vi "Periodic Tasks.vi"(8 "error in":errorcluster) -> ()   [LabVIEW 2015]
doc: "This VI runs in parallel to other tasks. It can contain as many user-defined periodic loops as you need. These can carry out PID or other sorts of timed response."
uses:
  <vilib>/Rock Robotics/WPI/PWM/Servo/WPI_ServoDeviceRef.ctl
  <vilib>/Rock Robotics/SystemInterfaces/DIO/FPGA_DIOPWMChannel.ctl
  <vilib>/Rock Robotics/WPI/PWM/WPI_PWMDeadband.ctl
  Team Code/IMU/LSM9DS1DevRef.ctl
  <vilib>/Rock Robotics/SystemInterfaces/i2clib/i2c_bus.ctl
  Team Code/IMU/Gyro_TypeDef.ctl
  Team Code/IMU/Accel_TypeDef.ctl
  Team Code/IMU/Mag_TypeDef.ctl
  Team Code/Periodic Task/Intake Enum..ctl
  Team Code/Periodic Task/Arm_defense_Type_Def.ctl
  Team Code/Periodic Task/Motor_Dir_Type_Def.ctl
  <vilib>/Rock Robotics/WPI/Solenoid/WPI_SolenoidValue.ctl
  <vilib>/Rock Robotics/WPI/MotorControl/WPI_MotorControlDeviceRef.ctl
  <vilib>/Rock Robotics/WPI/MotorControl/WPI_MotorControlType.ctl
  <vilib>/Rock Robotics/WPI/CAN/Jaguar/SubVIs/WPI_CANJaguar_ControlMode.ctl
  <vilib>/Rock Robotics/WPI/CAN/TalonSRX/WPI_CANTalonSRX_APIControlMode.ctl
  <vilib>/Rock Robotics/WPI/Solenoid/WPI_SolenoidDevRef.ctl
  <vilib>/Rock Robotics/WPI/Solenoid/WPI_SolenoidChannel.ctl
  Team Code/IMU/IMU_Global.vi
  Team Code/Global_Var/Drive_Global.vi
panel:
  out "Pitch":cluster{dbl, "Out":dbl, "Out":dbl}(graph)
  in  "Pitch_FIlt":dbl=0.1
  out "Waveform Chart":cluster{"Yaw":dbl, "Angle":dbl}(graph)
  in  "Quick_Turn":bool=TRUE
  in  "Reset":bool
  in  "PID Gains":T1
  in  "Drive_En_Reset":bool
  in  "auto_ds_en":bool
  in  "auto_us_en":bool
  in  "auto_us_spd":dbl=60000.0
  in  "auto_ds_spd_hiload":dbl
  in  "low_throt_thresh":dbl=20.0 format="%#_13g"
  in  "high_throt_thresh":dbl=75.0 format="%#_13g"
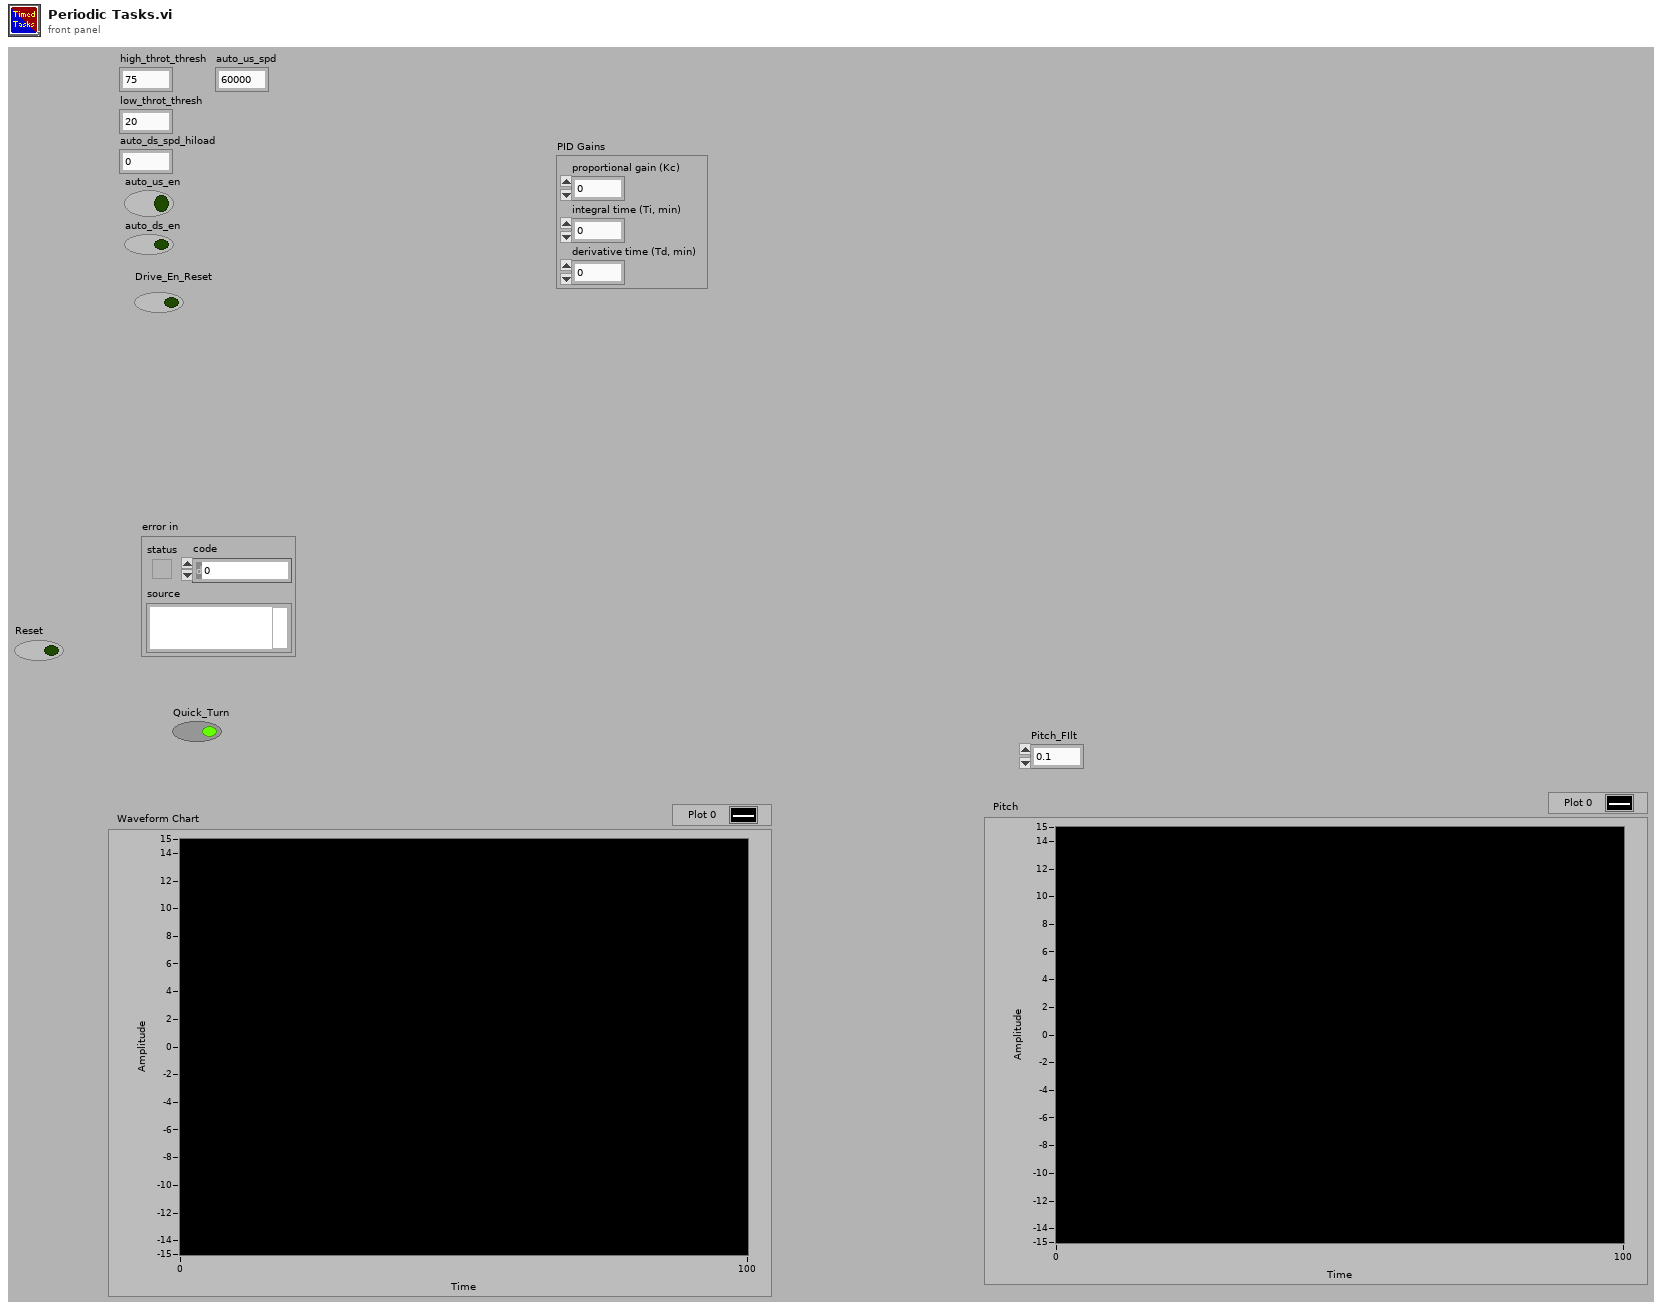
[diagram p1: front panel]
types:
  T1 = cluster{"proportional gain (Kc)":dbl, "integral time (Ti, min)":dbl, "derivative time (Td, min)":dbl}
  T2 = typedef "WPI_ServoDeviceRef.ctl" = cluster{"DeviceStatus":errorcluster, "PWM Channel":T3, "DeadBand":T4}
  T3 = typedef "FPGA_DIOPWMChannel.ctl" = enum8{"PWM 0", "PWM 1", "PWM 2", "PWM 3", "PWM 4", "PWM 5", "PWM 6", "PWM 7", "PWM 8", "PWM 9", "PWM MXP 0", "PWM MXP 1", "PWM MXP 2", "PWM MXP 3", "PWM MXP 4", "PWM MXP 5", "PWM MXP 6", "PWM MXP 7", "PWM MXP 8", "PWM MXP 9", "Invalid"}
  T4 = typedef "WPI_PWMDeadband.ctl" = cluster{"Name":string, "maxPositivePwm":i32, "minPositivePwm":i32, "centerPwm":i32, "maxNegativePwm":i32, "minNegativePwm":i32, "angularRange":u16}
  T5 = cluster{"ServoDeviceRef":T2, "error out":errorcluster}
  T6 = typedef "Motor_Type_Def.ctl" = cluster{"Drive_Motor":cluster{"RobotDriveDevRef":T7, "error out":errorcluster}, "Intake_1":cluster{"MotorControlDevRef":T8, "error out":errorcluster}, "Intake_Stage":cluster{"MotorControlDevRef":T8, "error out":errorcluster}, "Shooter_Motor_1":cluster{"MotorControlDevRef":T8, "error out":errorcluster}}
  T7 = typedef "WPI_RobotDriveDevRef.ctl" = cluster{"DevStatus":errorcluster, "Motors[]":T8[], "Square Inputs":bool, "Max Output":dbl}
  T8 = typedef "WPI_MotorControlDeviceRef.ctl" = cluster{"DeviceStatus":errorcluster, "Type":T9, "PWM":cluster{"PWM Channel":T3, "DeadBand":T4}, "CAN":cluster{"Device Number":u8, "Control Mode":T10, "Semaphore":T11, "Max Vout":dbl, "TalonSRX Control Mode":T12}, "Invert":bool}
  T9 = typedef "WPI_MotorControlType.ctl" = enum16{"PWM", "CAN", "CANTalonSRX"}
  T10 = typedef "WPI_CANJaguar_ControlMode.ctl" = enum8{"Percent VBus", "Current", "Speed", "Position", "Voltage"}
  T11 = typedef "Semaphore RefNum" = refnum<k1>
  T12 = typedef "WPI_CANTalonSRX_APIControlMode.ctl" = enum8{"Percent VBus", "Speed", "Position", "Slave", "Unchanged / Invalid", "Voltage Compensation", "Current", "Motion Profile"}
  T13 = typedef "Pneu_Type_Def.ctl" = cluster{"Intake_Arm":cluster{"SolenoidDevRef":T14, "error out":errorcluster}, "Gear":cluster{"SolenoidDevRef":T14, "error out":errorcluster}, "Flipper":cluster{"SolenoidDevRef":T14, "error out":errorcluster}, "Arm_defense":cluster{"SolenoidDevRef":T14, "error out":errorcluster}, "Compressor":cluster{"CompressorDevRef":T16, "error out":errorcluster}}
  T14 = typedef "WPI_SolenoidDevRef.ctl" = cluster{"DevStatus":errorcluster, "Pneumatics Control Module":u8, "Forward Solenoid Channel":T15, "Reverse Solenoid Channel":T15}
  T15 = typedef "WPI_SolenoidChannel.ctl" = enum8{"Solenoid 0", "Solenoid 1", "Solenoid 2", "Solenoid 3", "Solenoid 4", "Solenoid 5", "Solenoid 6", "Solenoid 7", "Invalid"}
  T16 = typedef "WPI_CompressorDevRef.ctl" = cluster{"DevStatus":errorcluster, "Pneumatics Control Module":u8}
  T17 = typedef "DIO_Type_Def.ctl" = cluster{"Left_Back":cluster{"SonarMB1010DigitalDevRef":T18, "error out":errorcluster}, "Left_Front":cluster{"SonarMB1010DigitalDevRef":T18, "error out":errorcluster}, "Right_Back":cluster{"SonarMB1010DigitalDevRef":T18, "error out":errorcluster}, "Right_Front":cluster{"SonarMB1010DigitalDevRef":T18, "error out":errorcluster}, "Front":cluster{"SonarMB1010DigitalDevRef":T18, "error out":errorcluster}, "Left Encoder":cluster{"EncoderDevRef":T21, "error out":errorcluster}, "Right Encoder":cluster{"EncoderDevRef":T21, "error out":errorcluster}, "Shooter Encoder":cluster{"CounterDevRef":T19, "error out":errorcluster}, "Intake_Storing":cluster{"DigitalInputDevRef":T24, "error out":errorcluster}, "Intake_Staged":cluster{"DigitalInputDevRef":T24, "error out":errorcluster}}
  T18 = typedef "WPI_SonarMB1010DigitalDeviceRef.ctl" = cluster{"CounterDevRef":T19, "Scaling factor (s/in)":dbl}
  T19 = typedef "WPI_CounterDevRef.ctl" = cluster{"DevStatus":errorcluster, "CntIndex":T20}
  T20 = typedef "FPGA_CounterCtrSystemIndex.ctl" = enum8{"Ctr 0", "Ctr 1", "Ctr 2", "Ctr 3", "Ctr 4", "Ctr 5", "Ctr 6", "Ctr 7", "Invalid"}
  T21 = typedef "WPI_EncoderDevRef.ctl" = cluster{"DevStatus":errorcluster, "EncoderIndex":T22, "CounterIndex":T20, "DistancePerCount":dbl, "Decoding Type":T23}
  T22 = typedef "FPGA_EncoderIdx.ctl" = enum8{"Enc 0", "Enc 1", "Enc 2", "Enc 3", "Enc 4", "Enc 5", "Enc 6", "Enc 7", "Invalid"}
  T23 = typedef "WPI_EncoderType.ctl" = enum16{"1x", "2x", "4x"}
  T24 = typedef "WPI_DigitalInputDevRef.ctl" = cluster{"DevStatus":errorcluster, "DIO Channel":T25}
  T25 = typedef "FPGA_DIOChannel.ctl" = enum8{"DIO 0", "DIO 1", "DIO 2", "DIO 3", "DIO 4", "DIO 5", "DIO 6", "DIO 7", "DIO 8", "DIO 9", "DIO MXP 0", "DIO MXP 1", "DIO MXP 2", "DIO MXP 3", "DIO MXP 4", "DIO MXP 5", "DIO MXP 6", "DIO MXP 7", "DIO MXP 8", "DIO MXP 9", "DIO MXP 10", "DIO MXP 11", "DIO MXP 12", "DIO MXP 13", "DIO MXP 14", "DIO MXP 15", "Invalid"}
  T26 = typedef "LSM9DS1DevRef.ctl" = cluster{"DevStatus":errorcluster, "Gyro Offset":cluster{"Xzero":dbl, "Yzero":dbl, "Zzero":dbl}, "StdDev Rates":cluster{"Xsdo":dbl, "Ysdo":dbl, "Zsdo":dbl}, "Reset":bool, "Accel Offset":cluster{"Xzero":dbl, "Yzero":dbl, "Zzero":dbl}, "Motion Thresh":dbl, "Mag Offset":cluster{"Xzero":dbl, "Yzero":dbl, "Zzero":dbl}, "I2C Bus":T27, "Handle":i32, "Anomaly Thresh":dbl, "Local Mag":dbl, "Accel/Gyro_Address":enum8{"0x6A", "0x6B"}, "Accel_Range":enum16{"±2g", "±16g", "±4g", "±8g", "disabled"}, "Gyro_Range":enum16{"±245dps", "±500dps", "disabled", "±2000dps"}, "Mag_Range":enum16{"±2 gauss", "±4 gauss", "±8 gauss", "±16 gauss", "disabled"}, "Mag_Address":enum8{"0x1C", "0x1E"}, "accel_active":bool, "gyro_active":bool, "mag_active":bool}
  T27 = typedef "i2c_bus.ctl" = enum16{"I2C On-Board", "I2C MXP", "Invalid"}
  T28 = typedef "WPI_GyroDevRef.ctl" = cluster{"DevStatus":errorcluster, "Analog Channel":T29, "Offset":dbl, "Gain (VoltsPerDegree/Second)":dbl, "Gyro Type":enum16{"Analog", "XRS450"}, "Handle":i32, "SPI Bus":T30, "Device Found":bool, "Sample Rate":dbl, "Calibrate On Open":bool}
  T29 = typedef "FPGA_AIChannel.ctl" = enum8{"AI 0", "AI 1", "AI 2", "AI 3", "AI MXP 0", "AI MXP 1", "AI MXP 2", "AI MXP 3", "Invalid"}
  T30 = typedef "spi_bus.ctl" = enum16{"SPI On-Board, CS0", "SPI On-Board, CS1", "SPI On-Board, CS2", "SPI On-Board, CS3", "SPI MXP", "Invalid"}
  T31 = typedef "WPI_AccelerometerDevRef.ctl" = cluster{"DevStatus":errorcluster, "Scaling":T32, "Analog Channels":T33, "I2C Bus":T27, "SPI Bus":T30, "Accel Range":T34, "ADXL Axes":T35, "Handle":i32, "Device Address":u8, "Accel Type":enum16{"Analog", "ADXL345 I2C", "ADXL345 SPI", "Internal", "ADXL362 SPI"}}
  T32 = typedef "WPI_AccelerometerScaling.ctl" = cluster{"Gain (VoltsPerG)":dbl, "Center Voltage":dbl}
  T33 = typedef "WPI_AccelerometerAnalogChannels.ctl" = cluster{"X-Axis":T29, "Y-Axis":T29, "Z-Axis":T29}
  T34 = typedef "ADXL345 Range.ctl" = u8
  T35 = typedef "WPI_AccelerometerADXL345 Axes.ctl" = cluster{"X-Axis":bool, "Y-Axis":bool, "Z-Axis":bool}
  T36 = cluster{"Auto_Aim":bool, "Auto_Aim_Enable":bool, "Shoot":bool, "Far_Shoot":bool}
  T37 = cluster{"Intake Arm Lowered":bool, "Motor Speed":dbl, "Rest_Encoder":bool, "Rest_Gyro":bool, "TeeterTotter Enable":bool, "Completed_Auto":bool}
  T38 = cluster{"Intake Arm Lowered":bool, "Motor Speed":dbl, "PortCullis_Enable":bool, "Rest_Encoder":bool, "Rest_Gyro":bool, "Completed_Auto":bool}
  T39 = cluster{"Motor Speed":dbl, "Rest_Encoder":bool, "Rest_Gyro":bool, "Rough Terrain On":bool, "Intake Arm Lowered":bool, "Completed_Auto":bool}
  T40 = cluster{"Drive_Enable":bool, "Auto_Aim":bool, "Intake Arm Lowered":bool, "Drive_FWD Speed":dbl, "One_Ball_Auto":bool, "Rest_Encoder":bool, "Rest_Gyro":bool, "Shoot":bool, "Stage":bool, "Angle_Setpoint":dbl}
  T41 = cluster{"Vision Distance":cluster{"1":dbl, "2":dbl, "3":dbl}, "Vision_angle":cluster{"1":dbl, "2":dbl, "3":dbl}, "Aimed?":bool}
  T42 = cluster{"Auto_Aim_Enable":bool, "CAM_Reset_IMU":bool, "Set_Point":dbl, "Aimed?":bool, "Enable_Cam":bool}
  T43 = typedef "Gyro_TypeDef.ctl" = cluster{"Pitch":dbl, "Yaw":dbl, "X Ang Rate":dbl, "Y Ang Rate":dbl, "Z Ang Rate":dbl, "Roll":dbl}
  T44 = typedef "Accel_TypeDef.ctl" = cluster{"X Accel":dbl, "Y Accel":dbl, "Z Accel":dbl, "Pitch":dbl, "Roll":dbl}
  T45 = typedef "Mag_TypeDef.ctl" = cluster{"X Mag":dbl, "Y Mag":dbl, "Z Mag":dbl}
  T46 = cluster{"LSM9DS1DevRef Out":T26, "Gyro":T43, "Accel":T44, "Mag":T45, "error out":errorcluster}
  T47 = cluster{"X-Axis":dbl, "Y-Axis":dbl, "Z-Axis":dbl}
  T48 = cluster{"Left_Back_Dist":dbl, "Left_Front_Dist":dbl, "Right_Back_Dist":dbl, "Right_Front_Dist":dbl, "Front_Dist":dbl, "Left_Dist":dbl, "Left_Angle":dbl, "Right_Dist":dbl, "Right_Angle":dbl}
  T49 = typedef "Auto_Selection.ctl" = enum16{"Low Bar", "Rough Terrain", "Rock Wall", "Ramparts", "Moat", "Cheval de Frise", "Portcullis", "None", "One  Ball", "Shoot"}
  T50 = cluster{"Auto_Selection":T49, "Auto_Enable":bool}
  T51 = cluster{"Right_En":cluster{"Distance":dbl, "Direction":bool, "Rate":dbl, "Stopped":bool}, "Left_En":cluster{"Distance":dbl, "Direction":bool, "Rate":dbl, "Stopped":bool}, "Shooter_En":cluster{"Distance":dbl, "Direction":bool, "Rate":dbl, "Stopped":bool}}
  T52 = typedef "WPI_DriverStationRobotMode2.ctl" = enum16{"Autonomous Disabled", "Autonomous Enabled", "Teleop Disabled", "Teleop Enabled", "Disconnected", "Finish", "Test Disabled", "Test Enabled", "Emergency Stopped"}
  T53 = typedef "WPI_CameraImageSize.ctl" = enum16{"640x480", "320x240", "160x120", "Custom"}
  T54 = cluster{"Climb":bool, "Close_Shot":bool, "Enable Vision":bool, "Far_Shot":bool, "Gear_Toggle":bool, "Intake":bool, "Left_Joystick_X":dbl, "Left_Joystick_Y":dbl, "Portcullis":bool, "Right_Joystick_X":dbl, "Right_Joystick_Y":dbl, "Robot Mode":T52, "image size":T53, "Speed Toggle":bool, "Intake Stage":bool, "Cheval":bool, "Intake_Motor_Man":dbl, "Stage_Motor_Man":dbl, "Lower_Intake_Arm":bool, "Lower_Intake_Def":bool, "Raise_Intake_Arm":bool, "Raise_Intake_Def":bool, "Flipper_Man":bool, "Auto_Aim":bool, "Low_Goal":bool}
  T55 = cluster{"Encoder_Var":cluster{"Right_En":cluster{"Distance":dbl, "Direction":bool, "Rate":dbl, "Stopped":bool}, "Left_En":cluster{"Distance":dbl, "Direction":bool, "Rate":dbl, "Stopped":bool}, "Shooter_En":cluster{"Distance":dbl, "Direction":bool, "Rate":dbl, "Stopped":bool}}, "JoyStick":cluster{"Climb":bool, "Close_Shot":bool, "Enable Vision":bool, "Far_Shot":bool, "Gear_Toggle":bool, "Intake":bool, "Left_Joystick_X":dbl, "Left_Joystick_Y":dbl, "Portcullis":bool, "Right_Joystick_X":dbl, "Right_Joystick_Y":dbl, "Robot Mode":T52, "image size":T53, "Speed Toggle":bool, "Intake Stage":bool, "Cheval":bool, "Intake_Motor_Man":dbl, "Stage_Motor_Man":dbl, "Lower_Intake_Arm":bool, "Lower_Intake_Def":bool, "Raise_Intake_Arm":bool, "Raise_Intake_Def":bool, "Flipper_Man":bool, "Auto_Aim":bool, "Low_Goal":bool}, "IMU":cluster{"LSM9DS1DevRef Out":T26, "Gyro":T43, "Accel":T44, "Mag":T45, "error out":errorcluster}, "Feedback":cluster{"Vision Distance":cluster{"1":dbl, "2":dbl, "3":dbl}, "Vision_angle":cluster{"1":dbl, "2":dbl, "3":dbl}, "Aimed?":bool}, "Ultar_Sonic":cluster{"Left_Back_Dist":dbl, "Left_Front_Dist":dbl, "Right_Back_Dist":dbl, "Right_Front_Dist":dbl, "Front_Dist":dbl, "Left_Dist":dbl, "Left_Angle":dbl, "Right_Dist":dbl, "Right_Angle":dbl}, "Auto_Contorl":cluster{"Auto_Selection":T49, "Auto_Enable":bool}}
  T56 = cluster{"Encoder_Var":cluster{"Right_En":cluster{"Distance":dbl, "Direction":bool, "Rate":dbl, "Stopped":bool}, "Left_En":cluster{"Distance":dbl, "Direction":bool, "Rate":dbl, "Stopped":bool}, "Shooter_En":cluster{"Distance":dbl, "Direction":bool, "Rate":dbl, "Stopped":bool}}, "JoyStick":cluster{"Climb":bool, "Close_Shot":bool, "Enable Vision":bool, "Far_Shot":bool, "Gear_Toggle":bool, "Intake":bool, "Left_Joystick_X":dbl, "Left_Joystick_Y":dbl, "Portcullis":bool, "Right_Joystick_X":dbl, "Right_Joystick_Y":dbl, "Robot Mode":T52, "image size":T53, "Speed Toggle":bool, "Intake Stage":bool, "Cheval":bool, "Intake_Motor_Man":dbl, "Stage_Motor_Man":dbl, "Lower_Intake_Arm":bool, "Lower_Intake_Def":bool, "Raise_Intake_Arm":bool, "Raise_Intake_Def":bool, "Flipper_Man":bool, "Auto_Aim":bool, "Low_Goal":bool}, "IMU":cluster{"LSM9DS1DevRef Out":T26, "Gyro":T43, "Accel":T44, "Mag":T45, "error out":errorcluster}, "Feedback":cluster{"Vision Distance":cluster{"1":dbl, "2":dbl, "3":dbl}, "Vision_angle":cluster{"1":dbl, "2":dbl, "3":dbl}, "Aimed?":bool}, "Ultar_Sonic":cluster{"Left_Back_Dist":dbl, "Left_Front_Dist":dbl, "Right_Back_Dist":dbl, "Right_Front_Dist":dbl, "Front_Dist":dbl, "Left_Dist":dbl, "Left_Angle":dbl, "Right_Dist":dbl, "Right_Angle":dbl}, "Rought_Ter":cluster{"Motor Speed":dbl, "Rest_Encoder":bool, "Rest_Gyro":bool, "Rough Terrain On":bool, "Intake Arm Lowered":bool, "Completed_Auto":bool}, "Portcullis":cluster{"Intake Arm Lowered":bool, "Motor Speed":dbl, "PortCullis_Enable":bool, "Rest_Encoder":bool, "Rest_Gyro":bool, "Completed_Auto":bool}, "One_Ball_Auto":cluster{"Drive_Enable":bool, "Auto_Aim":bool, "Intake Arm Lowered":bool, "Drive_FWD Speed":dbl, "One_Ball_Auto":bool, "Rest_Encoder":bool, "Rest_Gyro":bool, "Shoot":bool, "Stage":bool, "Angle_Setpoint":dbl}, "Teeter_Toter":cluster{"Intake Arm Lowered":bool, "Motor Speed":dbl, "Rest_Encoder":bool, "Rest_Gyro":bool, "TeeterTotter Enable":bool, "Completed_Auto":bool}, "Auto_Shoot":cluster{"Auto_Aim":bool, "Auto_Aim_Enable":bool, "Shoot":bool, "Far_Shoot":bool}}
  T57 = cluster{"Encoder_Var":cluster{"Right_En":cluster{"Distance":dbl, "Direction":bool, "Rate":dbl, "Stopped":bool}, "Left_En":cluster{"Distance":dbl, "Direction":bool, "Rate":dbl, "Stopped":bool}, "Shooter_En":cluster{"Distance":dbl, "Direction":bool, "Rate":dbl, "Stopped":bool}}, "JoyStick":cluster{"Climb":bool, "Close_Shot":bool, "Enable Vision":bool, "Far_Shot":bool, "Gear_Toggle":bool, "Intake":bool, "Left_Joystick_X":dbl, "Left_Joystick_Y":dbl, "Portcullis":bool, "Right_Joystick_X":dbl, "Right_Joystick_Y":dbl, "Robot Mode":T52, "image size":T53, "Speed Toggle":bool, "Intake Stage":bool, "Cheval":bool, "Intake_Motor_Man":dbl, "Stage_Motor_Man":dbl, "Lower_Intake_Arm":bool, "Lower_Intake_Def":bool, "Raise_Intake_Arm":bool, "Raise_Intake_Def":bool, "Flipper_Man":bool, "Auto_Aim":bool, "Low_Goal":bool}, "IMU":cluster{"LSM9DS1DevRef Out":T26, "Gyro":T43, "Accel":T44, "Mag":T45, "error out":errorcluster}, "Feedback":cluster{"Vision Distance":cluster{"1":dbl, "2":dbl, "3":dbl}, "Vision_angle":cluster{"1":dbl, "2":dbl, "3":dbl}, "Aimed?":bool}, "Ultar_Sonic":cluster{"Left_Back_Dist":dbl, "Left_Front_Dist":dbl, "Right_Back_Dist":dbl, "Right_Front_Dist":dbl, "Front_Dist":dbl, "Left_Dist":dbl, "Left_Angle":dbl, "Right_Dist":dbl, "Right_Angle":dbl}, "Rought_Ter":cluster{"Motor Speed":dbl, "Rest_Encoder":bool, "Rest_Gyro":bool, "Rough Terrain On":bool, "Intake Arm Lowered":bool, "Completed_Auto":bool}, "Portcullis":cluster{"Intake Arm Lowered":bool, "Motor Speed":dbl, "PortCullis_Enable":bool, "Rest_Encoder":bool, "Rest_Gyro":bool, "Completed_Auto":bool}, "One_Ball_Auto":cluster{"Drive_Enable":bool, "Auto_Aim":bool, "Intake Arm Lowered":bool, "Drive_FWD Speed":dbl, "One_Ball_Auto":bool, "Rest_Encoder":bool, "Rest_Gyro":bool, "Shoot":bool, "Stage":bool, "Angle_Setpoint":dbl}, "Teeter_Toter":cluster{"Intake Arm Lowered":bool, "Motor Speed":dbl, "Rest_Encoder":bool, "Rest_Gyro":bool, "TeeterTotter Enable":bool, "Completed_Auto":bool}, "AIM_Brain":cluster{"Auto_Aim_Enable":bool, "CAM_Reset_IMU":bool, "Set_Point":dbl, "Aimed?":bool, "Enable_Cam":bool}, "Auto_Shoot":cluster{"Auto_Aim":bool, "Auto_Aim_Enable":bool, "Shoot":bool, "Far_Shoot":bool}}
  T58 = cluster{"Encoder_Var":cluster{"Right_En":cluster{"Distance":dbl, "Direction":bool, "Rate":dbl, "Stopped":bool}, "Left_En":cluster{"Distance":dbl, "Direction":bool, "Rate":dbl, "Stopped":bool}, "Shooter_En":cluster{"Distance":dbl, "Direction":bool, "Rate":dbl, "Stopped":bool}}, "JoyStick":cluster{"Climb":bool, "Close_Shot":bool, "Enable Vision":bool, "Far_Shot":bool, "Gear_Toggle":bool, "Intake":bool, "Left_Joystick_X":dbl, "Left_Joystick_Y":dbl, "Portcullis":bool, "Right_Joystick_X":dbl, "Right_Joystick_Y":dbl, "Robot Mode":T52, "image size":T53, "Speed Toggle":bool, "Intake Stage":bool, "Cheval":bool, "Intake_Motor_Man":dbl, "Stage_Motor_Man":dbl, "Lower_Intake_Arm":bool, "Lower_Intake_Def":bool, "Raise_Intake_Arm":bool, "Raise_Intake_Def":bool, "Flipper_Man":bool, "Auto_Aim":bool, "Low_Goal":bool}, "IMU":cluster{"LSM9DS1DevRef Out":T26, "Gyro":T43, "Accel":T44, "Mag":T45, "error out":errorcluster}, "Feedback":cluster{"Vision Distance":cluster{"1":dbl, "2":dbl, "3":dbl}, "Vision_angle":cluster{"1":dbl, "2":dbl, "3":dbl}, "Aimed?":bool}, "Ultar_Sonic":cluster{"Left_Back_Dist":dbl, "Left_Front_Dist":dbl, "Right_Back_Dist":dbl, "Right_Front_Dist":dbl, "Front_Dist":dbl, "Left_Dist":dbl, "Left_Angle":dbl, "Right_Dist":dbl, "Right_Angle":dbl}, "Rought_Ter":cluster{"Motor Speed":dbl, "Rest_Encoder":bool, "Rest_Gyro":bool, "Rough Terrain On":bool, "Intake Arm Lowered":bool, "Completed_Auto":bool}, "Portcullis":cluster{"Intake Arm Lowered":bool, "Motor Speed":dbl, "PortCullis_Enable":bool, "Rest_Encoder":bool, "Rest_Gyro":bool, "Completed_Auto":bool}, "One_Ball_Auto":cluster{"Drive_Enable":bool, "Auto_Aim":bool, "Intake Arm Lowered":bool, "Drive_FWD Speed":dbl, "One_Ball_Auto":bool, "Rest_Encoder":bool, "Rest_Gyro":bool, "Shoot":bool, "Stage":bool, "Angle_Setpoint":dbl}, "Teeter_Toter":cluster{"Intake Arm Lowered":bool, "Motor Speed":dbl, "Rest_Encoder":bool, "Rest_Gyro":bool, "TeeterTotter Enable":bool, "Completed_Auto":bool}, "AIM_Brain":cluster{"Auto_Aim_Enable":bool, "CAM_Reset_IMU":bool, "Set_Point":dbl, "Aimed?":bool, "Enable_Cam":bool}, "Gear_Brain":cluster{"High_Gear_Cmd":bool}, "Setpoint_Arb":cluster{"Any True?":bool, "P Out":dbl}, "Drive":cluster{"Any True?":bool, "P Out":dbl}, "Auto_Shoot":cluster{"Auto_Aim":bool, "Auto_Aim_Enable":bool, "Shoot":bool, "Far_Shoot":bool}}
  T59 = cluster{"Climb_Motor_1":T8, "Climb_Motor_2":T8, "Climb_Pneu":T14}
  T60 = typedef "Arm_defense_Type_Def.ctl" = enum16{"Cheval de Frise", "Portcullis", "Out", "In", "Ball_Pickup"}
  T61 = typedef "WPI_SolenoidValue.ctl" = enum16{"Off", "On", "Forward", "Reverse"}
  T62 = cluster{"Gear Co mmand":T61, "Intake_Arm":T61, "Shooter_Arm":T61, "Flipper":T61}
  T63 = typedef "Motor_Dir_Type_Def.ctl" = enum16{"In", "Out", "Off"}
  T64 = cluster{"Shooter_Active":bool, "Stage_Motor":T63, "Shooter_Motor":dbl, "Shooter_Arm":T60}
  T65 = typedef "Intake Enum..ctl" = enum16{"Float", "Intake Portcullis", "Intake Ball Pickup", "Intake Cheval", " Intake Raised"}
  T66 = cluster{"Intake_Arm_Man_Act":bool, "Intake_Def_Man":T60, "Intake_Def_Man_Act":bool, "Intake_Motor_Man":T63, "Intake_Motor_Man_Act":bool, "Stage_Motor_Man":T63, "Stage_Motor_Man_Act":bool, "Flipper_Man":enum16{"Closed", "Open"}, "Flipper_Man_Act":bool, "Intake_Arm_Man":T65}
  T67 = cluster{"Intake_Motor_CMD":dbl, "Stage_Motor_CMD":dbl}
  T68 = cluster{"Intake Motor":T63, "Stage Motor":T63, "Flipper":enum16{"Closed", "Open"}, "Stage_Active":bool}
  T69 = cluster{"Intake_Motor":T63, "Intake_Position":T65, "Stage_Motor":T63, "Arm_Defense":T60, "Flipper":enum16{"Closed", "Open"}, "Intake_Active":bool}
  T70 = cluster{"Any True?":bool, "P_Out":enum16{"Closed", "Open"}}
  T71 = cluster{"Intake_Pos":T65, "Cheval_Active":bool, "Arm_Defense":T60}
  T72 = cluster{"Arm_Defense":T60, "Intake_Pos":T65, "Portcullis Active":bool}
  T73 = cluster{"Intake Storing":bool, "Intake_Stage":bool}
  T74 = cluster{"Ref_Num":cluster{"Motor":T6, "Pneu":T13, "DIO":T17}, "Ultar_Sonic":cluster{"Left_Back_Dist":dbl, "Left_Front_Dist":dbl, "Right_Back_Dist":dbl, "Right_Front_Dist":dbl, "Front_Dist":dbl, "Left_Dist":dbl, "Left_Angle":dbl, "Right_Dist":dbl, "Right_Angle":dbl}, "JoyStick":cluster{"Climb":bool, "Close_Shot":bool, "Enable Vision":bool, "Far_Shot":bool, "Gear_Toggle":bool, "Intake":bool, "Left_Joystick_X":dbl, "Left_Joystick_Y":dbl, "Portcullis":bool, "Right_Joystick_X":dbl, "Right_Joystick_Y":dbl, "Robot Mode":T52, "image size":T53, "Speed Toggle":bool, "Intake Stage":bool, "Cheval":bool, "Intake_Motor_Man":dbl, "Stage_Motor_Man":dbl, "Lower_Intake_Arm":bool, "Lower_Intake_Def":bool, "Raise_Intake_Arm":bool, "Raise_Intake_Def":bool, "Flipper_Man":bool, "Auto_Aim":bool, "Low_Goal":bool}, "Intake Var":cluster{"Intake Storing":bool, "Intake_Stage":bool}}
  T75 = cluster{"Ref_Num":cluster{"Motor":T6, "Pneu":T13, "DIO":T17}, "Ultar_Sonic":cluster{"Left_Back_Dist":dbl, "Left_Front_Dist":dbl, "Right_Back_Dist":dbl, "Right_Front_Dist":dbl, "Front_Dist":dbl, "Left_Dist":dbl, "Left_Angle":dbl, "Right_Dist":dbl, "Right_Angle":dbl}, "JoyStick":cluster{"Climb":bool, "Close_Shot":bool, "Enable Vision":bool, "Far_Shot":bool, "Gear_Toggle":bool, "Intake":bool, "Left_Joystick_X":dbl, "Left_Joystick_Y":dbl, "Portcullis":bool, "Right_Joystick_X":dbl, "Right_Joystick_Y":dbl, "Robot Mode":T52, "image size":T53, "Speed Toggle":bool, "Intake Stage":bool, "Cheval":bool, "Intake_Motor_Man":dbl, "Stage_Motor_Man":dbl, "Lower_Intake_Arm":bool, "Lower_Intake_Def":bool, "Raise_Intake_Arm":bool, "Raise_Intake_Def":bool, "Flipper_Man":bool, "Auto_Aim":bool, "Low_Goal":bool}, "Intake Var":cluster{"Intake Storing":bool, "Intake_Stage":bool}, "Intake_Brain":cluster{"Intake_Motor":T63, "Intake_Position":T65, "Stage_Motor":T63, "Arm_Defense":T60, "Flipper":enum16{"Closed", "Open"}, "Intake_Active":bool}, "Stage_Brain":cluster{"Intake Motor":T63, "Stage Motor":T63, "Flipper":enum16{"Closed", "Open"}, "Stage_Active":bool}, "Cheval_Brain":cluster{"Intake_Pos":T65, "Cheval_Active":bool, "Arm_Defense":T60}, "Shooter_Brain":cluster{"Shooter_Active":bool, "Stage_Motor":T63, "Shooter_Motor":dbl, "Shooter_Arm":T60}, "Port_Brain":cluster{"Arm_Defense":T60, "Intake_Pos":T65, "Portcullis Active":bool}, "Man":cluster{"Intake_Arm_Man_Act":bool, "Intake_Def_Man":T60, "Intake_Def_Man_Act":bool, "Intake_Motor_Man":T63, "Intake_Motor_Man_Act":bool, "Stage_Motor_Man":T63, "Stage_Motor_Man_Act":bool, "Flipper_Man":enum16{"Closed", "Open"}, "Flipper_Man_Act":bool, "Intake_Arm_Man":T65}}
  T76 = cluster{"Ref_Num":cluster{"Motor":T6, "Pneu":T13, "DIO":T17}, "Ultar_Sonic":cluster{"Left_Back_Dist":dbl, "Left_Front_Dist":dbl, "Right_Back_Dist":dbl, "Right_Front_Dist":dbl, "Front_Dist":dbl, "Left_Dist":dbl, "Left_Angle":dbl, "Right_Dist":dbl, "Right_Angle":dbl}, "JoyStick":cluster{"Climb":bool, "Close_Shot":bool, "Enable Vision":bool, "Far_Shot":bool, "Gear_Toggle":bool, "Intake":bool, "Left_Joystick_X":dbl, "Left_Joystick_Y":dbl, "Portcullis":bool, "Right_Joystick_X":dbl, "Right_Joystick_Y":dbl, "Robot Mode":T52, "image size":T53, "Speed Toggle":bool, "Intake Stage":bool, "Cheval":bool, "Intake_Motor_Man":dbl, "Stage_Motor_Man":dbl, "Lower_Intake_Arm":bool, "Lower_Intake_Def":bool, "Raise_Intake_Arm":bool, "Raise_Intake_Def":bool, "Flipper_Man":bool, "Auto_Aim":bool, "Low_Goal":bool}, "Intake Var":cluster{"Intake Storing":bool, "Intake_Stage":bool}, "Intake_Brain":cluster{"Intake_Motor":T63, "Intake_Position":T65, "Stage_Motor":T63, "Arm_Defense":T60, "Flipper":enum16{"Closed", "Open"}, "Intake_Active":bool}, "Stage_Brain":cluster{"Intake Motor":T63, "Stage Motor":T63, "Flipper":enum16{"Closed", "Open"}, "Stage_Active":bool}, "Cheval_Brain":cluster{"Intake_Pos":T65, "Cheval_Active":bool, "Arm_Defense":T60}, "Shooter_Brain":cluster{"Shooter_Active":bool, "Stage_Motor":T63, "Shooter_Motor":dbl, "Shooter_Arm":T60}, "Port_Brain":cluster{"Arm_Defense":T60, "Intake_Pos":T65, "Portcullis Active":bool}, "Man":cluster{"Intake_Arm_Man_Act":bool, "Intake_Def_Man":T60, "Intake_Def_Man_Act":bool, "Intake_Motor_Man":T63, "Intake_Motor_Man_Act":bool, "Stage_Motor_Man":T63, "Stage_Motor_Man_Act":bool, "Flipper_Man":enum16{"Closed", "Open"}, "Flipper_Man_Act":bool, "Intake_Arm_Man":T65}, "Intake_Pneu_arb":cluster{"Any True?":bool, "P Out":T65}, "Intake_Motor_Arb":cluster{"Any True?":bool, "P Out":T63}, "Stage_Motor_Arb":cluster{"Any True?":bool, "P Out":T63}, "Shooter Arm":cluster{"Any True?":bool, "P_Out":T60}, "Flipper_Arb":cluster{"Any True?":bool, "P_Out":enum16{"Closed", "Open"}}}
  T77 = cluster{"Ref_Num":cluster{"Motor":T6, "Pneu":T13, "DIO":T17}, "Ultar_Sonic":cluster{"Left_Back_Dist":dbl, "Left_Front_Dist":dbl, "Right_Back_Dist":dbl, "Right_Front_Dist":dbl, "Front_Dist":dbl, "Left_Dist":dbl, "Left_Angle":dbl, "Right_Dist":dbl, "Right_Angle":dbl}, "JoyStick":cluster{"Climb":bool, "Close_Shot":bool, "Enable Vision":bool, "Far_Shot":bool, "Gear_Toggle":bool, "Intake":bool, "Left_Joystick_X":dbl, "Left_Joystick_Y":dbl, "Portcullis":bool, "Right_Joystick_X":dbl, "Right_Joystick_Y":dbl, "Robot Mode":T52, "image size":T53, "Speed Toggle":bool, "Intake Stage":bool, "Cheval":bool, "Intake_Motor_Man":dbl, "Stage_Motor_Man":dbl, "Lower_Intake_Arm":bool, "Lower_Intake_Def":bool, "Raise_Intake_Arm":bool, "Raise_Intake_Def":bool, "Flipper_Man":bool, "Auto_Aim":bool, "Low_Goal":bool}, "Intake Var":cluster{"Intake Storing":bool, "Intake_Stage":bool}, "Intake_Brain":cluster{"Intake_Motor":T63, "Intake_Position":T65, "Stage_Motor":T63, "Arm_Defense":T60, "Flipper":enum16{"Closed", "Open"}, "Intake_Active":bool}, "Stage_Brain":cluster{"Intake Motor":T63, "Stage Motor":T63, "Flipper":enum16{"Closed", "Open"}, "Stage_Active":bool}, "Cheval_Brain":cluster{"Intake_Pos":T65, "Cheval_Active":bool, "Arm_Defense":T60}, "Shooter_Brain":cluster{"Shooter_Active":bool, "Stage_Motor":T63, "Shooter_Motor":dbl, "Shooter_Arm":T60}, "Port_Brain":cluster{"Arm_Defense":T60, "Intake_Pos":T65, "Portcullis Active":bool}, "Man":cluster{"Intake_Arm_Man_Act":bool, "Intake_Def_Man":T60, "Intake_Def_Man_Act":bool, "Intake_Motor_Man":T63, "Intake_Motor_Man_Act":bool, "Stage_Motor_Man":T63, "Stage_Motor_Man_Act":bool, "Flipper_Man":enum16{"Closed", "Open"}, "Flipper_Man_Act":bool, "Intake_Arm_Man":T65}, "Intake_Pneu_arb":cluster{"Any True?":bool, "P Out":T65}, "Intake_Motor_Arb":cluster{"Any True?":bool, "P Out":T63}, "Stage_Motor_Arb":cluster{"Any True?":bool, "P Out":T63}, "Shooter Arm":cluster{"Any True?":bool, "P_Out":T60}, "Flipper_Arb":cluster{"Any True?":bool, "P_Out":enum16{"Closed", "Open"}}, "Pneu_Cmd":cluster{"Gear Co mmand":T61, "Intake_Arm":T61, "Shooter_Arm":T61, "Flipper":T61}, "Motor_CMD":cluster{"Intake_Motor_CMD":dbl, "Stage_Motor_CMD":dbl}}
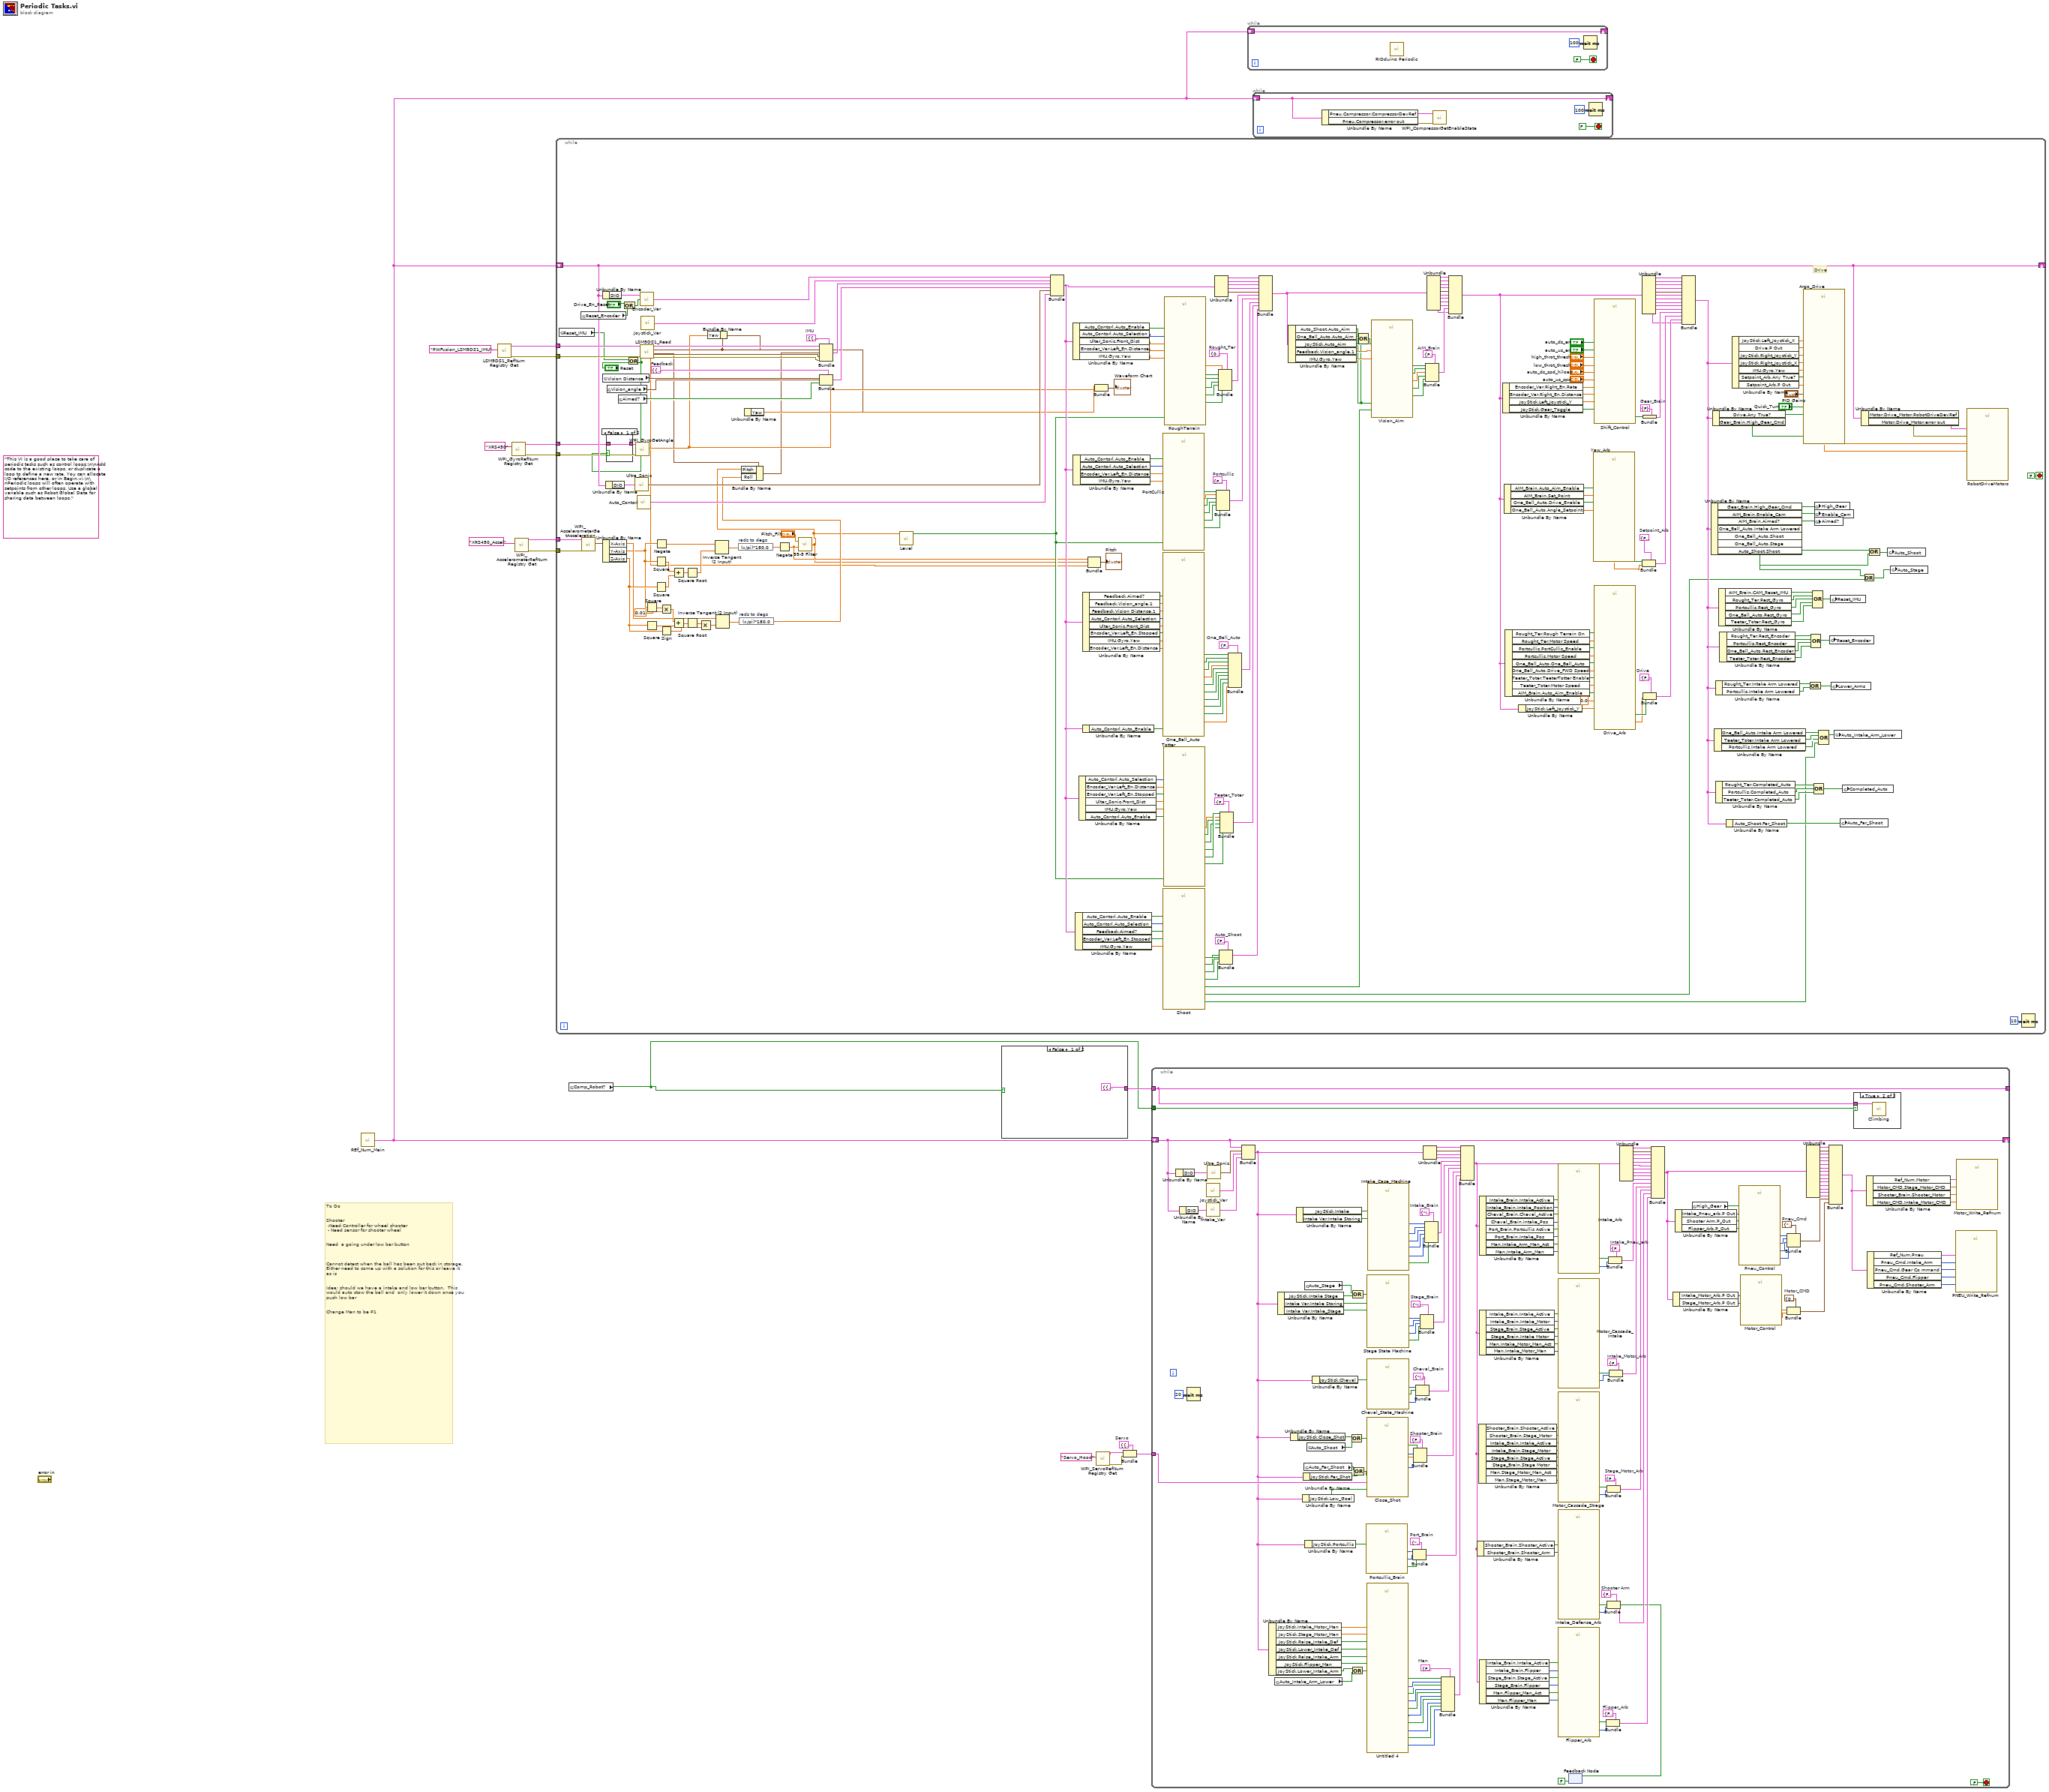
[diagram p0: block diagram]
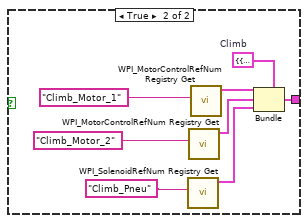
[diagram p2: hidden frame]
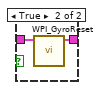
[diagram p4: hidden frame]
diagram:
  w9 = T5 {"ServoDeviceRef"={"DeviceStatus"={"status"=FALSE, "code"=0, "source"=""}, "PWM Channel"=enum."PWM 0", "DeadBand"={"Name"="", "maxPositivePwm"=0, "minPositivePwm"=0, "centerPwm"=0, "maxNegativePwm"=0, "minNegativePwm"=0, "angularRange"=0}}, "error out"={"status"=FALSE, "code"=0, "source"=""}}  # Servo
  (unwired) "This VI is a good place to take care of periodic tasks such as control loops.\n\nAdd code to the existing loops, or duplicate a loop to define a new rate. You can allocate I/O references here, or in Begin.vi.\n\nPeriodic loops will often operate with setpoints from other loops. Use a global variable such as Robot Global Data for sharing data between loops."
  # "To Do \n\n\nShooter\n -Need Controller for wheel shooter\n - Need sensor for shooter wheel\n\n\nNeed  a going under low bar button\n\n\n\nCannot detect when the ball has been put back in storage.  Either need to come up with a solution for this or leave it as is\n\n\nIdea: should we have a intake and low bar button.  This would auto stow the ball and  only lower it down once you push low bar \n\n\nChange Man to be P1"
  n1 = call "REf_Num_Main.vi"() -> ("Ref_Num"=w7:cluster{"Motor":T6, "Pneu":T13, "DIO":T17})
  n2 = call "LSM9DS1_RefNum Registry Get.vi"("refnum name"="PWFusion_LSM9DS1_IMU") -> ("error out"=w15:errorcluster, "LSM9DS1DevRef Out"=w16:T26)  [unwired: 9 in]
  n3 = call <vilib>:"WPI_GyroRefNum Registry Get.vi"("refnum name"="XRS450") -> ("error out"=w4:errorcluster, "GyroDevRef"=w5:T28)  [unwired: 9 in]
  n4 = call <vilib>:"WPI_AccelerometerRefNum Registry Get.vi"("refnum name"="XRS450_Accel") -> ("error out"=w1:errorcluster, "AccelerometerDevRef"=w2:T31)  [unwired: 9 in]
  n5 = while {
    shift-right: [w231] -> _
    shift-left: w7 -> [w231]
    tunnel: w16 -> [w276]
    tunnel: w15 -> [w275]
    tunnel: w5 -> [w64]
    tunnel: w4 -> [w60]
    tunnel: w2 -> [w55]
    tunnel: w1 -> [w54]
    stop <- FALSE stop-if-true
    w69 = T36 {"Auto_Aim"=FALSE, "Auto_Aim_Enable"=FALSE, "Shoot"=FALSE, "Far_Shoot"=FALSE}  # Auto_Shoot
    w75 = T37 {"Intake Arm Lowered"=FALSE, "Motor Speed"=0.0, "Rest_Encoder"=FALSE, "Rest_Gyro"=FALSE, "TeeterTotter Enable"=FALSE, "Completed_Auto"=FALSE}  # Teeter_Toter
    w77 = T38 {"Intake Arm Lowered"=FALSE, "Motor Speed"=0.0, "PortCullis_Enable"=FALSE, "Rest_Encoder"=FALSE, "Rest_Gyro"=FALSE, "Completed_Auto"=FALSE}  # Portcullis
    w79 = T39 {"Motor Speed"=0.0, "Rest_Encoder"=FALSE, "Rest_Gyro"=FALSE, "Rough Terrain On"=FALSE, "Intake Arm Lowered"=FALSE, "Completed_Auto"=FALSE}  # Rought_Ter
    w130 = T40 {"Drive_Enable"=FALSE, "Auto_Aim"=FALSE, "Intake Arm Lowered"=FALSE, "Drive_FWD Speed"=0.0, "One_Ball_Auto"=FALSE, "Rest_Encoder"=FALSE, "Rest_Gyro"=FALSE, "Shoot"=FALSE, "Stage"=FALSE, "Angle_Setpoint"=0.0}  # One_Ball_Auto
    w160 = T41 {"Vision Distance"={"1"=0.0, "2"=0.0, "3"=0.0}, "Vision_angle"={"1"=0.0, "2"=0.0, "3"=0.0}, "Aimed?"=FALSE}  # Feedback
    w168 = T42 {"Auto_Aim_Enable"=FALSE, "CAM_Reset_IMU"=FALSE, "Set_Point"=0.0, "Aimed?"=FALSE, "Enable_Cam"=FALSE}  # AIM_Brain
    w210 = cluster{"Any True?":bool, "P Out":dbl} {"Any True?"=FALSE, "P Out"=0.0}  # Drive
    w233 = cluster{"Any True?":bool, "P Out":dbl} {"Any True?"=FALSE, "P Out"=0.0}  # Setpoint_Arb
    w252 = cluster{"High_Gear_Cmd":bool} {"High_Gear_Cmd"=FALSE}  # Gear_Brain
    w259 = T46 {"LSM9DS1DevRef Out"={"DevStatus"={"status"=FALSE, "code"=0, "source"=""}, "Gyro Offset"={"Xzero"=0.0, "Yzero"=0.0, "Zzero"=0.0}, "StdDev Rates"={"Xsdo"=0.0, "Ysdo"=0.0, "Zsdo"=0.0}, "Reset"=FALSE, "Accel Offset"={"Xzero"=0.0, "Yzero"=0.0, "Zzero"=0.0}, "Motion Thresh"=0.0, "Mag Offset"={"Xzero"=0.0, "Yzero"=0.0, "Zzero"=0.0}, "I2C Bus"=enum."I2C On-Board", "Handle"=0, "Anomaly Thresh"=0.0, "Local Mag"=0.0, "Accel/Gyro_Address"=enum."0x6A", "Accel_Range"=enum."±2g", "Gyro_Range"=enum."±245dps", "Mag_Range"=enum."±2 gauss", "Mag_Address"=enum."0x1C", "accel_active"=FALSE, "gyro_active"=FALSE, "mag_active"=FALSE}, "Gyro"={"Pitch"=0.0, "Yaw"=0.0, "X Ang Rate"=0.0, "Y Ang Rate"=0.0, "Z Ang Rate"=0.0, "Roll"=0.0}, "Accel"={"X Accel"=0.0, "Y Accel"=0.0, "Z Accel"=0.0, "Pitch"=0.0, "Roll"=0.0}, "Mag"={"X Mag"=0.0, "Y Mag"=0.0, "Z Mag"=0.0}, "error out"={"status"=FALSE, "code"=0, "source"=""}}  # IMU
    # "Drive"
    n6 = global read "IMU_Global.vi" "Reset_IMU"() -> (w100:bool)
    n7 = global read "Drive_Global.vi" "Reset_Encoder"() -> (w215:bool)
    n8 = call <vilib>:"WPI_AccelerometerGetAcceleration.vi"("error in"=w54, "AccelerometerDevRef"=w55) -> ("Accelerations"=w37:T47)  [unwired: 7 in, 2 out]
    n9 = Unbundle By Name(w231) -> ("DIO"=w277:T17)
    n10 = Unbundle By Name(w37) -> ("X-Axis"=w31:dbl, "Y-Axis"=w30:dbl, "Z-Axis"=w36:dbl)
    n11 = global read "Drive_Global.vi" "Vision Distance"() -> (w164:cluster{"1":dbl, "2":dbl, "3":dbl})
    n12 = Unbundle By Name(w231) -> ("DIO"=w232:T17)
    n13 = global read "Drive_Global.vi" "Vision_angle"() -> (w163:cluster{"1":dbl, "2":dbl, "3":dbl})
    n14 = global read "Drive_Global.vi" "Aimed?"() -> (w161:bool)
    n15 = Compound Arithmetic op=OR("Drive_En_Reset", w215) -> (w214:bool)
    n16 = Or(x=w100, y="Reset") -> (x .or. y?=w58:bool)
    n17 = case shown="False" w58 {
      tunnel: [w283 w285] -> w65
      tunnel: w64 -> [w283 w284]
      frame False {
      }
      frame True {
        n18 = call <vilib>:"WPI_GyroReset.vi"("GyroDevRef"=w284) -> ("GyroDevRef"=w285:T28)  [unwired: 9 in, 1 out]
      }
    }
    n19 = call "Ultra_Sonic.vi"("output cluster 3"=w232) -> ("Ultar_Sonic"=w230:T48)
    n20 = call <vilib>:"WPI_GyroGetAngle.vi"("error in"=w60, "GyroDevRef"=w65) -> ("Angle"=w57:dbl)  [unwired: 5 in, 4 out]
    n21 = call "Auto_Contorl.vi"() -> ("Auto_Contorl"=w200:T50)
    n22 = call "Encoder_Var.vi"("Drive_En_Reset"=w214, "DIO"=w277) -> ("Encoder_Var"=w264:T51)  [unwired: 1 in]
    n23 = call "LSM9DS1_Read.vi"("LSM9DS1DevRef"=w276, "Reset"=w58, "error in (no error)"=w275) -> ("Filt_Pitch"=w24:dbl, "LSM9DS1DevRef Out"=w262:T26, "Gyro"=w27:T43, "Accel"=w26:T44, "Mag"=w261:T45, "error out"=w260:errorcluster)  [unwired: 7 in]
    n24 = call "Joystick_Var.vi"() -> ("JoyStick"=w263:T54)
    n25 = Square(x=w30) -> (x^2=w48:dbl)
    n26 = Square(x=w36) -> (x^2=w45:dbl)
    n27 = Square(x=w30) -> (x^2=w41:dbl)
    n28 = Square(x=w36) -> (x^2=w42:dbl)
    n29 = Negate(x=w30) -> (-x=w50:dbl)
    n30 = Multiply(x=w48, y=0.01 ("u 2")) -> (x*y=w49:dbl)
    n31 = Sign(1:w36) -> (0:w47:dbl)
    n32 = Add(x=w41, y=w42) -> (x+y=w43:dbl)
    n33 = Add(x=w49, y=w45) -> (x+y=w44:dbl)
    n34 = Square Root(x=w43) -> (sqrt(x)=w51:dbl)
    n35 = Square Root(x=w44) -> (sqrt(x)=w46:dbl)
    n36 = Multiply(x=w46, y=w47) -> (x*y=w52:dbl)
    n37 = Bundle By Name(cluster=w27, "Yaw"=w57) -> (w56:T43)
    n38 = Inverse Tangent (2 Input)(1:w51, 2:w50) -> (0:w39:dbl)
    n39 = Inverse Tangent (2 Input)(1:w52, 2:w31) -> (0:w40:dbl)
    n40 = expression code="(x/pi)*180.0" "rads to degs"(w39) -> (w38:dbl)
    n41 = expression code="(x/pi)*180.0" "rads to degs"(w40) -> (w35:dbl)
    n42 = Unbundle By Name(w27) -> ("Yaw"=w59:dbl)
    n43 = Negate(x=w38) -> (-x=w28:dbl)
    n44 = call "95-5 Filter.vi"("In"=w28, "Percent"="Pitch_FIlt") -> ("Out"=w23:dbl)
    n45 = Bundle By Name(cluster=w26, "Pitch"=w23, "Roll"=w35) -> (w34:T44)
    n46 = Bundle(cluster=w259, "LSM9DS1DevRef Out"=w262, "Gyro"=w56, "Accel"=w34, "Mag"=w261, "error out"=w260) -> (w62:T46)
    n47 = Bundle(cluster=w160, "Vision Distance"=w164, "Vision_angle"=w163, "Aimed?"=w161) -> (w162:T41)
    n48 = call "Level.vi"("In"=w23) -> ("Boolean"=w32:bool)  [unwired: 8 in]
    n49 = Bundle("Encoder_Var"=w264, "JoyStick"=w263, "IMU"=w62, "Feedback"=w162, "Ultar_Sonic"=w230, "Auto_Contorl"=w200) -> (w94:T55)  [unwired: 1 in]
    n50 = Unbundle By Name(w94) -> ("Auto_Contorl.Auto_Enable"=w199:bool, "Auto_Contorl.Auto_Selection"=w198:T49, "Ultar_Sonic.Front_Dist"=w229:dbl, "Encoder_Var.Left_En.Distance"=w228:dbl, "IMU.Gyro.Yaw"=w227:dbl)
    n51 = Unbundle By Name(w94) -> ("Auto_Contorl.Auto_Enable"=w197:bool, "Auto_Contorl.Auto_Selection"=w196:T49, "Encoder_Var.Left_En.Distance"=w195:dbl, "IMU.Gyro.Yaw"=w194:dbl)
    n52 = Unbundle By Name(w94) -> ("Auto_Contorl.Auto_Enable"=w93:bool, "Auto_Contorl.Auto_Selection"=w92:T49, "Feedback.Aimed?"=w91:bool, "Encoder_Var.Left_En.Stopped"=w90:bool, "IMU.Gyro.Yaw"=w89:dbl)
    n53 = Unbundle By Name(w94) -> ("Auto_Contorl.Auto_Selection"=w121:T49, "Encoder_Var.Left_En.Distance"=w120:dbl, "Encoder_Var.Left_En.Stopped"=w119:bool, "Ultar_Sonic.Front_Dist"=w118:dbl, "IMU.Gyro.Yaw"=w117:dbl, "Auto_Contorl.Auto_Enable"=w97:bool)
    n54 = Unbundle By Name(w94) -> ("Feedback.Aimed?"=w158:bool, "Feedback.Vision_angle.1"=w165:dbl, "Feedback.Vision Distance.1"=w159:dbl, "Auto_Contorl.Auto_Selection"=w157:T49, "Ultar_Sonic.Front_Dist"=w156:dbl, "Encoder_Var.Left_En.Stopped"=w155:bool, "IMU.Gyro.Yaw"=w154:dbl, "Encoder_Var.Left_En.Distance"=w153:dbl)
    n55 = Unbundle By Name(w94) -> ("Auto_Contorl.Auto_Enable"=w96:bool)
    n56 = Bundle(w28, "Out"=w23, "Filt_Pitch"=w24) -> (→"Pitch":cluster{dbl, "Out":dbl, "Filt_Pitch":dbl})  [unwired: 1 in]
    n57 = Bundle("Yaw"=w59, "Angle"=w57) -> (→"Waveform Chart":cluster{"Yaw":dbl, "Angle":dbl})  [unwired: 1 in]
    n58 = call "PortCullis.vi"("Level"=w32, "Auto_Enable"=w197, "Auto_Selection"=w196, "Yaw"=w194, "Encoder"=w195) -> ("Rest_Encoder"=w190:bool, "Intake Arm Lowered"=w193:bool, "PortCullis_Enable"=w191:bool, "Motor Speed"=w192:dbl, "Completed_Auto"=w78:bool, "Rest_Gyro"=w189:bool)  [unwired: 1 in]
    n59 = call "One_Ball_Auto.vi"("Cam_Angle_To_Target"=w165, "Stopped"=w155, "Dist to target"=w159, "Auto_Control"=w157, "Encoder_Left"=w153, "Ultra_Sonic_Dist"=w156, "Auto_Enable"=w96, "Yaw"=w154, "Aimed?"=w158) -> ("Intake Arm Lowered"=w150:bool, "Drive_FWD Speed"=w149:dbl, "Angle_Setpoint"=w143:dbl, "Stage"=w144:bool, "Drive_Enable"=w152:bool, "Shoot"=w145:bool, "Auto_Aim"=w151:bool, "Rest_Encoder"=w147:bool, "Rest_Gyro"=w146:bool, "One_Ball_Auto"=w148:bool)  [unwired: 9 in]
    n60 = call "Shoot.vi"("Auto_Enable"=w93, "Aimed?"=w91, "Stopped?"=w90, "Yaw"=w89, "Auto_Selection"=w92) -> ("Far_Shoot"=w70:bool, "Hunt"=w19:bool, "Shoot"=w86:bool, "Auto_Aim"=w88:bool, "Lower_Arm"=w18:bool, "Auto_Aim_Enable"=w87:bool, "Stage"=w20:bool)
    n61 = call "Totter.vi"("Ultra_Sonic_Dist"=w118, "Level"=w32, "Encoder"=w120, "Auto_Enable"=w97, "Yaw"=w117, "Auto_Selection"=w121, "Stopped"=w119) -> ("Rest_Gyro"=w113:bool, "TeeterTotter Enable"=w112:bool, "Intake Arm Lowered"=w116:bool, "Motor Speed"=w115:dbl, "Rest_Encoder"=w114:bool, "Completed_Auto"=w76:bool)  [unwired: 3 in]
    n62 = call "RoughTerrain.vi"("Auto_Selection"=w198, "Auto_Enable"=w199, "Dist_Foward"=w229, "Level"=w32, "Encoder"=w228, "Yaw"=w227) -> ("Rough Terrain On"=w202:bool, "Rest_Encoder"=w204:bool, "Rest_Gyro"=w203:bool, "Completed_Auto"=w66:bool, "Motor Speed"=w205:dbl, "Intake Arm Lowered"=w201:bool)  [unwired: 4 in]
    n63 = Unbundle(w94) -> ("Encoder_Var"=w226:T51, "JoyStick"=w225:T54, "IMU"=w224:T46, "Feedback"=w223:T41, "Ultar_Sonic"=w222:T48)  [unwired: 1 out]
    n64 = Bundle(cluster=w77, "Intake Arm Lowered"=w193, "Motor Speed"=w192, "PortCullis_Enable"=w191, "Rest_Encoder"=w190, "Rest_Gyro"=w189, "Completed_Auto"=w78) -> (w186:T38)
    n65 = Bundle(cluster=w79, "Motor Speed"=w205, "Rest_Encoder"=w204, "Rest_Gyro"=w203, "Rough Terrain On"=w202, "Intake Arm Lowered"=w201, "Completed_Auto"=w66) -> (w187:T39)
    n66 = Bundle(cluster=w69, "Auto_Aim"=w88, "Auto_Aim_Enable"=w87, "Shoot"=w86, "Far_Shoot"=w70) -> (w85:T36)
    n67 = Bundle(cluster=w75, "Intake Arm Lowered"=w116, "Motor Speed"=w115, "Rest_Encoder"=w114, "Rest_Gyro"=w113, "TeeterTotter Enable"=w112, "Completed_Auto"=w76) -> (w141:T37)
    n68 = Bundle(cluster=w130, "Drive_Enable"=w152, "Auto_Aim"=w151, "Intake Arm Lowered"=w150, "Drive_FWD Speed"=w149, "One_Ball_Auto"=w148, "Rest_Encoder"=w147, "Rest_Gyro"=w146, "Shoot"=w145, "Stage"=w144, "Angle_Setpoint"=w143) -> (w142:T40)
    n69 = Bundle("Encoder_Var"=w226, "JoyStick"=w225, "IMU"=w224, "Feedback"=w223, "Ultar_Sonic"=w222, "Rought_Ter"=w187, "Portcullis"=w186, "One_Ball_Auto"=w142, "Teeter_Toter"=w141, "Auto_Shoot"=w85) -> (w221:T56)  [unwired: 1 in]
    n70 = Unbundle By Name(w221) -> ("Auto_Shoot.Auto_Aim"=w29:bool, "One_Ball_Auto.Auto_Aim"=w129:bool, "JoyStick.Auto_Aim"=w128:bool, "Feedback.Vision_angle.1"=w238:dbl, "IMU.Gyro.Yaw"=w167:dbl)
    n71 = Compound Arithmetic op=OR(w29, w129, w128) -> (w127:bool)
    n72 = call "Vision_Aim.vi"("Cam_Angle"=w238, "Yaw"=w167, "Auto_Aim"=w127, "Auto_Shoot_Aim"=w29, "Hunt"=w19) -> ("Aimed?"=w170:bool, "Auto_Aim_Enable"=w173:bool, "Enable_Cam"=w169:bool, "Set_Point"=w171:dbl, "CAM_Reset_IMU"=w172:bool)  [unwired: 1 in]
    n73 = Bundle(cluster=w168, "Auto_Aim_Enable"=w173, "CAM_Reset_IMU"=w172, "Set_Point"=w171, "Aimed?"=w170, "Enable_Cam"=w169) -> (w138:T42)
    n74 = Unbundle(w221) -> ("Encoder_Var"=w256:T51, "JoyStick"=w255:T54, "IMU"=w254:T46, "Feedback"=w242:T41, "Ultar_Sonic"=w220:T48, "Rought_Ter"=w219:T39, "Portcullis"=w188:T38, "One_Ball_Auto"=w140:T40, "Teeter_Toter"=w139:T37, "Auto_Shoot"=w84:T36)
    n75 = Bundle("Encoder_Var"=w256, "JoyStick"=w255, "IMU"=w254, "Feedback"=w242, "Ultar_Sonic"=w220, "Rought_Ter"=w219, "Portcullis"=w188, "One_Ball_Auto"=w140, "Teeter_Toter"=w139, "AIM_Brain"=w138, "Auto_Shoot"=w84) -> (w207:T57)  [unwired: 1 in]
    n76 = Unbundle By Name(w207) -> ("Encoder_Var.Right_En.Rate"=w258:dbl, "Encoder_Var.Right_En.Distance"=w257:dbl, "JoyStick.Left_Joystick_Y"=w266:dbl, "JoyStick.Gear_Toggle"=w265:bool)
    n77 = Unbundle By Name(w207) -> ("AIM_Brain.Auto_Aim_Enable"=w237:bool, "AIM_Brain.Set_Point"=w236:dbl, "One_Ball_Auto.Drive_Enable"=w123:bool, "One_Ball_Auto.Angle_Setpoint"=w122:dbl)
    n78 = Unbundle By Name(w207) -> ("Rought_Ter.Rough Terrain On"=w212:bool, "Rought_Ter.Motor Speed"=w213:dbl, "Portcullis.PortCullis_Enable"=w182:bool, "Portcullis.Motor Speed"=w181:dbl, "One_Ball_Auto.One_Ball_Auto"=w132:bool, "One_Ball_Auto.Drive_FWD Speed"=w131:dbl, "Teeter_Toter.TeeterTotter Enable"=w108:bool, "Teeter_Toter.Motor Speed"=w107:dbl, "AIM_Brain.Auto_Aim_Enable"=w103:bool)
    n79 = Unbundle By Name(w207) -> ("JoyStick.Left_Joystick_Y"=w101:dbl)
    n80 = call "Yaw_Arb.vi"("P1_Value"=w236, "P1_Enable"=w237, "P2_Value"=w122, "P2_Enable"=w123) -> ("P Out"=w234:dbl, "Any True?"=w235:bool)  [unwired: 10 in]
    n81 = call "Shift_Control.vi"("right_whlspd"=w257, "left_whlspd"=w258, "Joystick_Y"=w266, "high_throt_thresh"="high_throt_thresh", "low_throt_thresh"="low_throt_thresh", "auto_ds_spd_hiload"="auto_ds_spd_hiload", "auto_us_en"="auto_us_en", "auto_us_spd"="auto_us_spd", "auto_ds_en"="auto_ds_en", "manual_shift_req"=w265) -> ("High_Gear_Cmd"=w253:bool)  [unwired: 9 in]
    n82 = call "Drive_Arb.vi"("P1_Value"=w213, "P1_Enable"=w212, "P3_Enable"=w132, "P5_Value"=0.0, "P2_Value"=w181, "P3_Value"=w131, "P4_Value"=w107, "Default"=w101, "P2_Enable"=w182, "P4_Enable"=w108, "P5_Enable"=w103) -> ("P Out"=w206:dbl, "Any True?"=w211:bool)  [unwired: 3 in]
    n83 = Unbundle(w207) -> ("Encoder_Var"=w247:T51, "JoyStick"=w246:T54, "IMU"=w245:T46, "Feedback"=w244:T41, "Ultar_Sonic"=w241:T48, "Rought_Ter"=w185:T39, "Portcullis"=w184:T38, "One_Ball_Auto"=w183:T40, "Teeter_Toter"=w137:T37, "AIM_Brain"=w136:T42, "Auto_Shoot"=w83:T36)
    n84 = Bundle(cluster=w233, "Any True?"=w235, "P Out"=w234) -> (w134:cluster{"Any True?":bool, "P Out":dbl})
    n85 = Bundle(cluster=w210, "Any True?"=w211, "P Out"=w206) -> (w133:cluster{"Any True?":bool, "P Out":dbl})
    n86 = Bundle(cluster=w252, "High_Gear_Cmd"=w253) -> (w135:cluster{"High_Gear_Cmd":bool})
    n87 = Bundle("Encoder_Var"=w247, "JoyStick"=w246, "IMU"=w245, "Feedback"=w244, "Ultar_Sonic"=w241, "Rought_Ter"=w185, "Portcullis"=w184, "One_Ball_Auto"=w183, "Teeter_Toter"=w137, "AIM_Brain"=w136, "Gear_Brain"=w135, "Setpoint_Arb"=w134, "Drive"=w133, "Auto_Shoot"=w83) -> (w68:T58)  [unwired: 1 in]
    n88 = Unbundle By Name(w68) -> ("Gear_Brain.High_Gear_Cmd"=w243:bool, "AIM_Brain.Enable_Cam"=w240:bool, "AIM_Brain.Aimed?"=w166:bool, "One_Ball_Auto.Shoot"=w82:bool, "One_Ball_Auto.Stage"=w22:bool, "Auto_Shoot.Shoot"=w81:bool)  [unwired: 1 out]
    n89 = Unbundle By Name(w68) -> ("Drive.Any True?"=w99:bool, "Gear_Brain.High_Gear_Cmd"=w98:bool)
    n90 = Unbundle By Name(w68) -> ("One_Ball_Auto.Intake Arm Lowered"=w111:bool, "Teeter_Toter.Intake Arm Lowered"=w110:bool, "Portcullis.Intake Arm Lowered"=w95:bool)
    n91 = Unbundle By Name(w68) -> ("Rought_Ter.Intake Arm Lowered"=w175:bool, "Portcullis.Intake Arm Lowered"=w174:bool)
    n92 = Unbundle By Name(w68) -> ("Rought_Ter.Completed_Auto"=w74:bool, "Portcullis.Completed_Auto"=w73:bool, "Teeter_Toter.Completed_Auto"=w72:bool)
    n93 = Unbundle By Name(w68) -> ("AIM_Brain.CAM_Reset_IMU"=w218:bool, "Rought_Ter.Rest_Gyro"=w217:bool, "Portcullis.Rest_Gyro"=w180:bool, "One_Ball_Auto.Rest_Gyro"=w125:bool, "Teeter_Toter.Rest_Gyro"=w105:bool)
    n94 = Unbundle By Name(w68) -> ("Rought_Ter.Rest_Encoder"=w178:bool, "Portcullis.Rest_Encoder"=w177:bool, "One_Ball_Auto.Rest_Encoder"=w126:bool, "Teeter_Toter.Rest_Encoder"=w106:bool)
    n95 = Unbundle By Name(w68) -> ("Auto_Shoot.Far_Shoot"=w67:bool)
    n96 = Unbundle By Name(w68) -> ("JoyStick.Left_Joystick_X"=w251:dbl, "Drive.P Out"=w250:dbl, "JoyStick.Right_Joystick_Y"=w249:dbl, "JoyStick.Right_Joystick_X"=w248:dbl, "IMU.Gyro.Yaw"=w239:dbl, "Setpoint_Arb.Any True?"=w209:bool, "Setpoint_Arb.P Out"=w208:dbl)
    n97 = call "Argo_Drive.vi"("Speed_Main"=w250, "Speed_Limit"=w251, "Turning_Limit"=w249, "Turning_PID_Enable"=w209, "PID Gains"="PID Gains", "Turning_Main"=w248, "Auto_Enable"=w99, "High_Gear"=w98, "Quick_Turn"="Quick_Turn", "Turning_Setpoint"=w208, "Yaw"=w239) -> ("Left_Motor"=w274:dbl, "Right_Motor"=w273:dbl)  [unwired: 7 in]
    n98 = Compound Arithmetic op=OR(w175, w174) -> (w176:bool)
    n99 = Compound Arithmetic op=OR(w178, w177, w126, w106) -> (w179:bool)
    n100 = Compound Arithmetic op=OR(w218, w217, w180, w125, w105) -> (w124:bool)
    n101 = Compound Arithmetic op=OR(w74, w73, w72) -> (w71:bool)
    n102 = global write "Drive_Global.vi" "High_Gear"(w243) -> ()
    n103 = global write "Drive_Global.vi" "Enable_Cam"(w240) -> ()
    n104 = global write "Drive_Global.vi" "Aimed?"(w166) -> ()
    n105 = Compound Arithmetic op=OR(w111, w110, w95, w18) -> (w109:bool)
    n106 = global write "Drive_Global.vi" "Reset_Encoder"(w179) -> ()
    n107 = global write "IMU_Global.vi" "Reset_IMU"(w124) -> ()
    n108 = global write "Drive_Global.vi" "Lower_Arms"(w176) -> ()
    n109 = global write "Drive_Global.vi" "Auto_Intake_Arm_Lower"(w109) -> ()
    n110 = global write "Drive_Global.vi" "Auto_Far_Shoot"(w67) -> ()
    n111 = global write "Drive_Global.vi" "Completed_Auto"(w71) -> ()
    n112 = Unbundle By Name(w231) -> ("Motor.Drive_Motor.RobotDriveDevRef"=w280:T7, "Motor.Drive_Motor.error out"=w279:errorcluster)
    n113 = Or(x=w22, y=w20) -> (x .or. y?=w21:bool)
    n114 = Compound Arithmetic op=OR(w82, w81) -> (w80:bool)
    n115 = global write "Drive_Global.vi" "Auto_Shoot"(w80) -> ()
    n116 = global write "Drive_Global.vi" "Auto_Stage"(w21) -> ()
    n117 = call "RobotDriveMotors.vi"("error in (no error)"=w279, "RightSpeed"=w273, "LeftSpeed"=w274, "RobotDriveDevRef"=w280) -> ()  [unwired: 5 in, 3 out]
    n118 = Wait (ms)(milliseconds to wait=u32 10) -> ()  [unwired: 1 out]
  }
  n119 = global read "Drive_Global.vi" "Comp_Robot?"() -> (w13:bool)
  n120 = case shown="False" w13 {
    tunnel: [T59 {"Climb_Motor_1"={"DeviceStatus"={"status"=FALSE, "code"=0, "source"=""}, "Type"=enum."PWM", "PWM"={"PWM Channel"=enum."PWM 0", "DeadBand"={"Name"="", "maxPositivePwm"=0, "minPositivePwm"=0, "centerPwm"=0, "maxNegativePwm"=0, "minNegativePwm"=0, "angularRange"=0}}, "CAN"={"Device Number"=0, "Control Mode"=enum."Percent VBus", "Semaphore"=refnum, "Max Vout"=0.0, "TalonSRX Control Mode"=enum."Percent VBus"}, "Invert"=FALSE}, "Climb_Motor_2"={"DeviceStatus"={"status"=FALSE, "code"=0, "source"=""}, "Type"=enum."PWM", "PWM"={"PWM Channel"=enum."PWM 0", "DeadBand"={"Name"="", "maxPositivePwm"=0, "minPositivePwm"=0, "centerPwm"=0, "maxNegativePwm"=0, "minNegativePwm"=0, "angularRange"=0}}, "CAN"={"Device Number"=0, "Control Mode"=enum."Percent VBus", "Semaphore"=refnum, "Max Vout"=0.0, "TalonSRX Control Mode"=enum."Percent VBus"}, "Invert"=FALSE}, "Climb_Pneu"={"DevStatus"={"status"=FALSE, "code"=0, "source"=""}, "Pneumatics Control Module"=0, "Forward Solenoid Channel"=enum."Solenoid 0", "Reverse Solenoid Channel"=enum."Solenoid 0"}} ("Climb") w288] -> w14
    frame False {
    }
    frame True {
      w287 = T59 {"Climb_Motor_1"={"DeviceStatus"={"status"=FALSE, "code"=0, "source"=""}, "Type"=enum."PWM", "PWM"={"PWM Channel"=enum."PWM 0", "DeadBand"={"Name"="", "maxPositivePwm"=0, "minPositivePwm"=0, "centerPwm"=0, "maxNegativePwm"=0, "minNegativePwm"=0, "angularRange"=0}}, "CAN"={"Device Number"=0, "Control Mode"=enum."Percent VBus", "Semaphore"=refnum, "Max Vout"=0.0, "TalonSRX Control Mode"=enum."Percent VBus"}, "Invert"=FALSE}, "Climb_Motor_2"={"DeviceStatus"={"status"=FALSE, "code"=0, "source"=""}, "Type"=enum."PWM", "PWM"={"PWM Channel"=enum."PWM 0", "DeadBand"={"Name"="", "maxPositivePwm"=0, "minPositivePwm"=0, "centerPwm"=0, "maxNegativePwm"=0, "minNegativePwm"=0, "angularRange"=0}}, "CAN"={"Device Number"=0, "Control Mode"=enum."Percent VBus", "Semaphore"=refnum, "Max Vout"=0.0, "TalonSRX Control Mode"=enum."Percent VBus"}, "Invert"=FALSE}, "Climb_Pneu"={"DevStatus"={"status"=FALSE, "code"=0, "source"=""}, "Pneumatics Control Module"=0, "Forward Solenoid Channel"=enum."Solenoid 0", "Reverse Solenoid Channel"=enum."Solenoid 0"}}  # Climb
      n121 = call <vilib>:"WPI_SolenoidRefNum Registry Get.vi"("refnum name"="Climb_Pneu") -> ("SolenoidDevRef"=w289:T14)  [unwired: 9 in, 1 out]
      n122 = call <vilib>:"WPI_MotorControlRefNum Registry Get.vi"("refnum name"="Climb_Motor_2") -> ("MotorControlDevRef"=w290:T8)  [unwired: 9 in, 1 out]
      n123 = call <vilib>:"WPI_MotorControlRefNum Registry Get.vi"("refnum name"="Climb_Motor_1") -> ("MotorControlDevRef"=w291:T8)  [unwired: 9 in, 1 out]
      n124 = Bundle(cluster=w287, "Climb_Motor_1"=w291, "Climb_Motor_2"=w290, "Climb_Pneu"=w289) -> (w288:T59)
    }
  }
  n125 = call <vilib>:"WPI_ServoRefNum Registry Get.vi"("refnum name"="Servo_Hood") -> ("error out"=w10:errorcluster, "ServoDeviceRef"=w11:T2)  [unwired: 9 in]
  n126 = Bundle(cluster=w9, "ServoDeviceRef"=w11, "error out"=w10) -> (w8:T5)
  n127 = while {
    shift-right: [w474] -> _
    shift-left: w7 -> [w474]
    tunnel: w14 -> [w304]
    tunnel: [w304] -> _
    tunnel: w13 -> [w303]
    tunnel: w8 -> [w302]
    stop <- FALSE stop-if-true
    w305 = cluster{"Any True?":bool, "P_Out":T60} {"Any True?"=FALSE, "P_Out"=enum."Cheval de Frise"}  # Shooter Arm
    w307 = T62 {"Gear Co mmand"=enum."Off", "Intake_Arm"=enum."Off", "Shooter_Arm"=enum."Off", "Flipper"=enum."Off"}  # Pneu_Cmd
    w310 = T64 {"Shooter_Active"=FALSE, "Stage_Motor"=enum."In", "Shooter_Motor"=0.0, "Shooter_Arm"=enum."Cheval de Frise"}  # Shooter_Brain
    w326 = T66 {"Intake_Arm_Man_Act"=FALSE, "Intake_Def_Man"=enum."Cheval de Frise", "Intake_Def_Man_Act"=FALSE, "Intake_Motor_Man"=enum."In", "Intake_Motor_Man_Act"=FALSE, "Stage_Motor_Man"=enum."In", "Stage_Motor_Man_Act"=FALSE, "Flipper_Man"=enum."Closed", "Flipper_Man_Act"=FALSE, "Intake_Arm_Man"=enum."Intake Portcullis"}  # Man
    w371 = T67 {"Intake_Motor_CMD"=0.0, "Stage_Motor_CMD"=0.0}  # Motor_CMD
    w375 = cluster{"Any True?":bool, "P Out":T63} {"Any True?"=FALSE, "P Out"=enum."In"}  # Stage_Motor_Arb
    w377 = cluster{"Any True?":bool, "P Out":T63} {"Any True?"=FALSE, "P Out"=enum."In"}  # Intake_Motor_Arb
    w378 = T68 {"Intake Motor"=enum."In", "Stage Motor"=enum."In", "Flipper"=enum."Closed", "Stage_Active"=FALSE}  # Stage_Brain
    w379 = T69 {"Intake_Motor"=enum."In", "Intake_Position"=enum."Intake Portcullis", "Stage_Motor"=enum."In", "Arm_Defense"=enum."Cheval de Frise", "Flipper"=enum."Closed", "Intake_Active"=FALSE}  # Intake_Brain
    w388 = T70 {"Any True?"=FALSE, "P_Out"=enum."Closed"}  # Flipper_Arb
    w396 = T71 {"Intake_Pos"=enum."Intake Portcullis", "Cheval_Active"=FALSE, "Arm_Defense"=enum."Cheval de Frise"}  # Cheval_Brain
    w401 = T72 {"Arm_Defense"=enum."Cheval de Frise", "Intake_Pos"=enum."Intake Portcullis", "Portcullis Active"=FALSE}  # Port_Brain
    w440 = cluster{"Any True?":bool, "P Out":T65} {"Any True?"=FALSE, "P Out"=enum."Intake Portcullis"}  # Intake_Pneu_arb
    n128 = Unbundle By Name(w474) -> ("DIO"=w479:T17)
    n129 = Unbundle By Name(w474) -> ("DIO"=w475:T17)
    n130 = Wait (ms)(milliseconds to wait=u32 20) -> ()  [unwired: 1 out]
    n131 = call "Intake_Var.vi"("DIO"=w475) -> ("Intake Var"=w473:T73)
    n132 = call "Joystick_Var.vi"() -> ("JoyStick"=w477:T54)
    n133 = call "Ultra_Sonic.vi"("output cluster 3"=w479) -> ("Ultar_Sonic"=w478:T48)
    n134 = Bundle("Ref_Num"=w474, "Ultar_Sonic"=w478, "JoyStick"=w477, "Intake Var"=w473) -> (w299:T74)  [unwired: 1 in]
    n135 = Unbundle By Name(w299) -> ("JoyStick.Intake_Motor_Man"=w363:dbl, "JoyStick.Stage_Motor_Man"=w362:dbl, "JoyStick.Raise_Intake_Def"=w361:bool, "JoyStick.Lower_Intake_Def"=w360:bool, "JoyStick.Raise_Intake_Arm"=w359:bool, "JoyStick.Flipper_Man"=w323:bool, "JoyStick.Lower_Intake_Arm"=w321:bool)
    n136 = global read "Drive_Global.vi" "Auto_Intake_Arm_Lower"() -> (w320:bool)
    n137 = Unbundle By Name(w299) -> ("JoyStick.Intake Stage"=w315:bool, "Intake Var.Intake Storing"=w316:bool, "Intake Var.Intake_Stage"=w471:bool)
    n138 = Unbundle By Name(w299) -> ("JoyStick.Close_Shot"=w319:bool)
    n139 = Unbundle By Name(w299) -> ("JoyStick.Intake"=w476:bool, "Intake Var.Intake Storing"=w472:bool)
    n140 = Unbundle By Name(w299) -> ("JoyStick.Low_Goal"=w298:bool)
    n141 = Unbundle By Name(w299) -> ("JoyStick.Far_Shot"=w296:bool)
    n142 = global read "Drive_Global.vi" "Auto_Far_Shoot"() -> (w297:bool)
    n143 = global read "Drive_Global.vi" "Auto_Stage"() -> (w313:bool)
    n144 = Unbundle By Name(w299) -> ("JoyStick.Portcullis"=w364:bool)
    n145 = global read "Drive_Global.vi" "Auto_Shoot"() -> (w318:bool)
    n146 = Unbundle By Name(w299) -> ("JoyStick.Cheval"=w445:bool)
    n147 = Compound Arithmetic op=OR(w319, w318) -> (w317:bool)
    n148 = Compound Arithmetic op=OR(w321, w320) -> (w322:bool)
    n149 = Compound Arithmetic op=OR(w313, w315) -> (w314:bool)
    n150 = Compound Arithmetic op=OR(w297, w296) -> (w295:bool)
    n151 = call "Portcullis_Brain.vi"("Portcullis Enable"=w364) -> ("Portcullis Active"=w402:bool, "Intake_Pos"=w403:T65, "Arm_Defense"=w404:T60)
    n152 = call "Close_Shot.vi"("Far Shot"=w295, "Low_Goal"=w298, "Servo_Ref"=w302, "Close_Shot"=w317) -> ("Shooter_Motor"=w369:dbl, "Shooter_Arm"=w311:T60, "Stage_Motor"=w370:T63, "Shooter_Active"=w368:bool)  [unwired: 1 in]
    n153 = call "Untitled 4.vi"("Lower_Intake_Man"=w322, "Raise_Intake_Man"=w359, "Flipper_Man"=w323, "Lower_Intake_Def"=w360, "Raise_Intake_Def"=w361, "Intake_Motor_Man"=w363, "Stage_Motor_Man"=w362) -> ("Flipper_Man"=w329:enum16{"Closed", "Open"}, "Flipper_Man_Act"=w328:bool, "Intake_Arm_Man"=w327:T65, "Intake_Arm_Man_Act"=w336:bool, "Intake_Def_Man"=w335:T60, "Intake_Def_Man_Act"=w334:bool, "Intake_Motor_Man_Act"=w332:bool, "Stage_Motor_Man_Act"=w330:bool, "Stage_Motor_Man"=w331:T63, "Intake_Motor_Man"=w333:T63)  [unwired: 3 in]
    n154 = call "Stage State Machine.vi"("Stage Button"=w314, "Stage Sensor"=w471, "Intake Sensor"=w316) -> ("Stage Motor"=w466:T63, "Intake Motor"=w467:T63, "Flipper"=w413:enum16{"Closed", "Open"}, "Stage_Active"=w409:bool)
    n155 = call "Cheval_State_Machine.vi"("Cheval_Button"=w445) -> ("Arm_Defense"=w397:T60, "Cheval_Active"=w407:bool, "Intake_Pos"=w447:T65)  [unwired: 8 in]
    n156 = call "Intake_Case_Machine.vi"("Intake_Sensor"=w472, "Intake_Button"=w476) -> ("Intake_Active"=w408:bool, "Arm_Defense"=w415:T60, "Intake_Motor"=w470:T63, "Stage_Motor"=w468:T63, "Intake_Position"=w469:T65, "Flipper"=w414:enum16{"Closed", "Open"})  [unwired: 1 in]
    n157 = Bundle(cluster=w401, "Arm_Defense"=w404, "Intake_Pos"=w403, "Portcullis Active"=w402) -> (w400:T72)
    n158 = Bundle(cluster=w310, "Shooter_Active"=w368, "Stage_Motor"=w370, "Shooter_Motor"=w369, "Shooter_Arm"=w311) -> (w412:T64)
    n159 = Bundle(cluster=w396, "Intake_Pos"=w447, "Cheval_Active"=w407, "Arm_Defense"=w397) -> (w446:T71)
    n160 = Bundle(cluster=w378, "Intake Motor"=w467, "Stage Motor"=w466, "Flipper"=w413, "Stage_Active"=w409) -> (w460:T68)
    n161 = Unbundle(w299) -> ("Ref_Num"=w465:cluster{"Motor":T6, "Pneu":T13, "DIO":T17}, "Ultar_Sonic"=w464:T48, "JoyStick"=w463:T54, "Intake Var"=w462:T73)
    n162 = Bundle(cluster=w379, "Intake_Motor"=w470, "Intake_Position"=w469, "Stage_Motor"=w468, "Arm_Defense"=w415, "Flipper"=w414, "Intake_Active"=w408) -> (w461:T69)
    n163 = Bundle(cluster=w326, "Intake_Arm_Man_Act"=w336, "Intake_Def_Man"=w335, "Intake_Def_Man_Act"=w334, "Intake_Motor_Man"=w333, "Intake_Motor_Man_Act"=w332, "Stage_Motor_Man"=w331, "Stage_Motor_Man_Act"=w330, "Flipper_Man"=w329, "Flipper_Man_Act"=w328, "Intake_Arm_Man"=w327) -> (w358:T66)
    n164 = Bundle("Ref_Num"=w465, "Ultar_Sonic"=w464, "JoyStick"=w463, "Intake Var"=w462, "Intake_Brain"=w461, "Stage_Brain"=w460, "Cheval_Brain"=w446, "Shooter_Brain"=w412, "Port_Brain"=w400, "Man"=w358) -> (w395:T75)  [unwired: 1 in]
    n165 = Unbundle By Name(w395) -> ("Shooter_Brain.Shooter_Active"=w309:bool, "Shooter_Brain.Shooter_Arm"=w308:T60)
    n166 = Unbundle By Name(w395) -> ("Shooter_Brain.Shooter_Active"=w451:bool, "Shooter_Brain.Stage_Motor"=w450:T63, "Intake_Brain.Intake_Active"=w448:bool, "Intake_Brain.Stage_Motor"=w449:T63, "Stage_Brain.Stage_Active"=w406:bool, "Stage_Brain.Stage Motor"=w405:T63, "Man.Stage_Motor_Man_Act"=w340:bool, "Man.Stage_Motor_Man"=w339:T63)
    n167 = Unbundle By Name(w395) -> ("Intake_Brain.Intake_Active"=w457:bool, "Intake_Brain.Intake_Position"=w456:T65, "Cheval_Brain.Cheval_Active"=w444:bool, "Cheval_Brain.Intake_Pos"=w443:T65, "Port_Brain.Portcullis Active"=w399:bool, "Port_Brain.Intake_Pos"=w398:T65, "Man.Intake_Arm_Man_Act"=w343:bool, "Man.Intake_Arm_Man"=w344:T65)
    n168 = Unbundle By Name(w395) -> ("Intake_Brain.Intake_Active"=w455:bool, "Intake_Brain.Intake_Motor"=w454:T63, "Stage_Brain.Stage_Active"=w453:bool, "Stage_Brain.Intake Motor"=w452:T63, "Man.Intake_Motor_Man_Act"=w342:bool, "Man.Intake_Motor_Man"=w341:T63)
    n169 = Unbundle By Name(w395) -> ("Intake_Brain.Intake_Active"=w394:bool, "Intake_Brain.Flipper"=w393:enum16{"Closed", "Open"}, "Stage_Brain.Stage_Active"=w392:bool, "Stage_Brain.Flipper"=w391:enum16{"Closed", "Open"}, "Man.Flipper_Man_Act"=w325:bool, "Man.Flipper_Man"=w324:enum16{"Closed", "Open"})
    n170 = call "Intake_Arb.vi"("P1_Value"=w456, "P1_Enable"=w457, "P3_Enable"=w399, "P2_Value"=w443, "P3_Value"=w398, "P4_Value"=w344, "P2_Enable"=w444, "P4_Enable"=w343) -> ("P Out"=w441:T65, "Any True?"=w442:bool)  [unwired: 6 in]
    n171 = call "Motor_Cascade_Intake.vi"("P1_Value"=w454, "P1_Enable"=w455, "P3_Enable"=w342, "P2_Value"=w452, "P3_Value"=w341, "P2_Enable"=w453) -> ("P Out"=w431:T63, "Any True?"=w432:bool)  [unwired: 8 in]
    n172 = call "Motor_Cascade_Strage.vi"("P1_Value"=w450, "P1_Enable"=w451, "P3_Enable"=w406, "P2_Value"=w449, "P3_Value"=w405, "P4_Value"=w339, "P2_Enable"=w448, "P4_Enable"=w340) -> ("P Out"=w430:T63, "Any True?"=w376:bool)  [unwired: 6 in]
    n173 = call "Intake_Defense_Arb.vi"("P1_Value"=w308, "P1_Enable"=w309) -> ("Any True?"=w301:bool, "P_Out"=w306:T60)  [unwired: 12 in]
    n174 = call "Flipper_Arb.vi"("P1_Value"=w393, "P1_Enable"=w394, "P3_Enable"=w325, "P2_Value"=w391, "P3_Value"=w324, "P2_Enable"=w392) -> ("P_Out"=w389:enum16{"Closed", "Open"}, "Any True?"=w390:bool)  [unwired: 8 in]
    n175 = feedback-in #1(w301) -> ()
    n176 = feedback #1(FALSE ("Any True?")) -> ()  [unwired: 1 in]
    n177 = Bundle(cluster=w388, "Any True?"=w390, "P_Out"=w389) -> (w351:T70)
    n178 = Bundle(cluster=w375, "Any True?"=w376, "P Out"=w430) -> (w353:cluster{"Any True?":bool, "P Out":T63})
    n179 = Bundle(cluster=w305, "Any True?"=w301, "P_Out"=w306) -> (w352:cluster{"Any True?":bool, "P_Out":T60})
    n180 = Bundle(cluster=w440, "Any True?"=w442, "P Out"=w441) -> (w355:cluster{"Any True?":bool, "P Out":T65})
    n181 = Bundle(cluster=w377, "Any True?"=w432, "P Out"=w431) -> (w354:cluster{"Any True?":bool, "P Out":T63})
    n182 = Unbundle(w395) -> ("Ref_Num"=w439:cluster{"Motor":T6, "Pneu":T13, "DIO":T17}, "Ultar_Sonic"=w438:T48, "JoyStick"=w437:T54, "Intake Var"=w436:T73, "Intake_Brain"=w435:T69, "Stage_Brain"=w434:T68, "Cheval_Brain"=w433:T71, "Shooter_Brain"=w411:T64, "Port_Brain"=w357:T72, "Man"=w356:T66)
    n183 = Bundle("Ref_Num"=w439, "Ultar_Sonic"=w438, "JoyStick"=w437, "Intake Var"=w436, "Intake_Brain"=w435, "Stage_Brain"=w434, "Cheval_Brain"=w433, "Shooter_Brain"=w411, "Port_Brain"=w357, "Man"=w356, "Intake_Pneu_arb"=w355, "Intake_Motor_Arb"=w354, "Stage_Motor_Arb"=w353, "Shooter Arm"=w352, "Flipper_Arb"=w351) -> (w374:T76)  [unwired: 1 in]
    n184 = Unbundle By Name(w374) -> ("Intake_Motor_Arb.P Out"=w338:T63, "Stage_Motor_Arb.P Out"=w337:T63)
    n185 = Unbundle By Name(w374) -> ("Intake_Pneu_arb.P Out"=w429:T65, "Shooter Arm.P_Out"=w387:T60, "Flipper_Arb.P_Out"=w386:enum16{"Closed", "Open"})
    n186 = global read "Drive_Global.vi" "High_Gear"() -> (w312:bool)
    n187 = call "Pneu_Control.vi"("Shooter_Arm"=w387, "Flipper_Arb"=w386, "Gear"=w312, "Intake Arm"=w429) -> ("Gear Co mmand"=w385:T61, "Flipper"=w382:T61, "Shooter_Arm"=w383:T61, "Intake_Arm"=w384:T61)
    n188 = call "Motor_Control.vi"("Stage_Motor"=w337, "Intake_Motor"=w338) -> ("Stage_Motor_CMD"=w372:dbl, "Intake_Motor_CMD"=w373:dbl)  [unwired: 8 in]
    n189 = Bundle(cluster=w307, "Gear Co mmand"=w385, "Intake_Arm"=w384, "Shooter_Arm"=w383, "Flipper"=w382) -> (w346:T62)
    n190 = Bundle(cluster=w371, "Intake_Motor_CMD"=w373, "Stage_Motor_CMD"=w372) -> (w345:T67)
    n191 = Unbundle(w374) -> ("Ref_Num"=w428:cluster{"Motor":T6, "Pneu":T13, "DIO":T17}, "Ultar_Sonic"=w427:T48, "JoyStick"=w426:T54, "Intake Var"=w425:T73, "Intake_Brain"=w424:T69, "Stage_Brain"=w423:T68, "Cheval_Brain"=w422:T71, "Shooter_Brain"=w421:T64, "Port_Brain"=w420:T72, "Man"=w419:T66, "Intake_Pneu_arb"=w410:cluster{"Any True?":bool, "P Out":T65}, "Intake_Motor_Arb"=w350:cluster{"Any True?":bool, "P Out":T63}, "Stage_Motor_Arb"=w349:cluster{"Any True?":bool, "P Out":T63}, "Shooter Arm"=w348:cluster{"Any True?":bool, "P_Out":T60}, "Flipper_Arb"=w347:T70)
    n192 = Bundle("Ref_Num"=w428, "Ultar_Sonic"=w427, "JoyStick"=w426, "Intake Var"=w425, "Intake_Brain"=w424, "Stage_Brain"=w423, "Cheval_Brain"=w422, "Shooter_Brain"=w421, "Port_Brain"=w420, "Man"=w419, "Intake_Pneu_arb"=w410, "Intake_Motor_Arb"=w350, "Stage_Motor_Arb"=w349, "Shooter Arm"=w348, "Flipper_Arb"=w347, "Pneu_Cmd"=w346, "Motor_CMD"=w345) -> (w418:T77)  [unwired: 1 in]
    n193 = case shown="True" w303 {
      tunnel: w304 -> [_ w482]
      frame False {
      }
      frame True {
        n194 = call "Climbing.vi"("Climb in"=w482) -> ()  [unwired: 11 in]
      }
    }
    n195 = Unbundle By Name(w418) -> ("Ref_Num.Motor"=w459:T6, "Motor_CMD.Stage_Motor_CMD"=w367:dbl, "Shooter_Brain.Shooter_Motor"=w366:dbl, "Motor_CMD.Intake_Motor_CMD"=w365:dbl)
    n196 = Unbundle By Name(w418) -> ("Ref_Num.Pneu"=w458:T13, "Pneu_Cmd.Intake_Arm"=w417:T61, "Pneu_Cmd.Gear Co mmand"=w416:T61, "Pneu_Cmd.Flipper"=w381:T61, "Pneu_Cmd.Shooter_Arm"=w380:T61)
    n197 = call "PNEU_Write_Refnum.vi"("Shooter_Arm"=w380, "Flipper"=w381, "Gear"=w416, "Intake_Arm"=w417, "Pneu"=w458) -> ()  [unwired: 7 in]
    n198 = call "Motor_Write_Refnum.vi"("Motor_Dev_Ref"=w459, "Shooter_Motor_1"=w366, "Intake_Stage"=w367, "Intake_1"=w365) -> ()  [unwired: 8 in]
  }
  n199 = while {
    shift-right: [w483] -> _
    shift-left: w7 -> [w483]
    stop <- FALSE stop-if-true
    n200 = call "RIOduino Periodic.vi"() -> ()  [unwired: 12 in]
    n201 = Wait (ms)(milliseconds to wait=u32 100) -> ()  [unwired: 1 out]
  }
  n202 = while {
    shift-right: [w486] -> _
    shift-left: w7 -> [w486]
    stop <- FALSE stop-if-true
    n203 = Unbundle By Name(w486) -> ("Pneu.Compressor.CompressorDevRef"=w488:T16, "Pneu.Compressor.error out"=w487:errorcluster)
    n204 = call <vilib>:"WPI_CompressorGetEnableState.vi"("error in (no error)"=w487, "CompressorDevRef"=w488) -> ()  [unwired: 6 in, 4 out]
    n205 = Wait (ms)(milliseconds to wait=u32 100) -> ()  [unwired: 1 out]
  }
